vi "复材超声C扫缺陷分析评定软件.vi"() -> ()   [LabVIEW 2018]
doc: "使用该模板构建用户界面事件处理设计模式。将模板应用于对话框及其它用户界面。用户也可创建并执行VI可按照与用户界面事件相同方式处理的用户定义事件。"
uses:
  <vilib>/Utility/NIReport.llb/Report Type.ctl
  <vilib>/addons/_office/_exclsub.llb/font.ctl
  <vilib>/Utility/NIReport.llb/HTML Report Image Alignment.ctl
  <vilib>/Utility/NIReport.llb/Append Report Text (str wrap).vi
  <vilib>/Utility/NIReport.llb/Append Image to Report (path wrap).vi
  <vilib>/addons/_office/word.llb/Word Easy Table (str).vi
  <vilib>/Utility/NIReport.llb/NI_report.lvclass
  <vilib>/vision/NI_Vision_Development_Module.lvlib
  <vilib>/Utility/NIReport.llb/Word/NI_Word.lvclass
  <vilib>/addons/_office/NI_ReportGenerationToolkit.lvlib
  <vilib>/Utility/NIReport.llb/NI_ReportGenerationCore.lvlib
panel:
  in  "删除完成 2":bool caption="定量分析"
  in  "标注完成":bool caption="定量分析"
  in  "删除标注":bool caption="定量分析"
  out "输入的灰度阈值":dbl caption="值"
  out "反射图原始路径":path
  out "穿透图原始路径":path
  out "ROImask":T1(plugin-control)
  in  "Operation 2":enum16{"overlay rectangle"}(ring)
  out "模式选择":u16(ring) items=["只读穿透图", "穿透图和反射图结合"]
  out "添加的路径":path
  out "连接的字符串 2":string
  out "临界面积百分比值":dbl
  out "临界Z值":i32
  out "标注后的图片路径":path
  out "弥散类检测结果合并":string[][](table)
  out "分层类检测结果合并":string[][](table)
  out "弥散类检测结果":string[][](table)
  out "分层类检测结果":string[][](table)
  out "部位信息":string[](array[string])=["", "34.500000", "32.500000", "1121", "34", "54.955926", "分层类", "不合格", ""]
  out "连接的字符串":string
  in  "完成标注":bool caption="定量分析"
  out "框数":dbl
  in  "Operation":enum16{"overlay rectangle"}(ring)
  out "自定义字体":T2={"Desired Font (Application)"=enum."Application Font", "[User-specified Font]"={"Font Name"="", "Size"=12, "Strikeout?"=FALSE, "Italic?"=FALSE, "Underline?"=FALSE, "Outline?"=FALSE, "Shadow?"=FALSE, "Bold?"=FALSE, "Rotation Angle"=0.0}, "Horizontal Alignment"=0, "Vertical Alignment"=0} {"Horizontal Alignment" items=["Left", "Center", "Right"]; "Vertical Alignment" items=["Bottom", "Top", "Baseline"]}
  out "框组":T3(array[cluster])
  out "质量等级":string
  out "灰度阈值":dbl
  in  "stop":bool caption="停止"
  in  "导入图像":bool caption="导入图片"
  in  "图像预处理":bool
  in  "自定义色彩":bool
  in  "开始标注":bool caption="定量分析"
  in  "查看标注":bool caption="辅助定性分析"
  in  "生成评定结果":bool caption="生成原始记录"
  in  "?":enum32{"穿透图", "反射图"}(tab)
  out "穿透图":T1(plugin-control)
  out "反射图":T1(plugin-control)
  out "产品规格":cluster{"产品长度（周长）（mm）":dbl, "产品宽度（母线长）（mm）":dbl}
  out "图像分辨率":T4
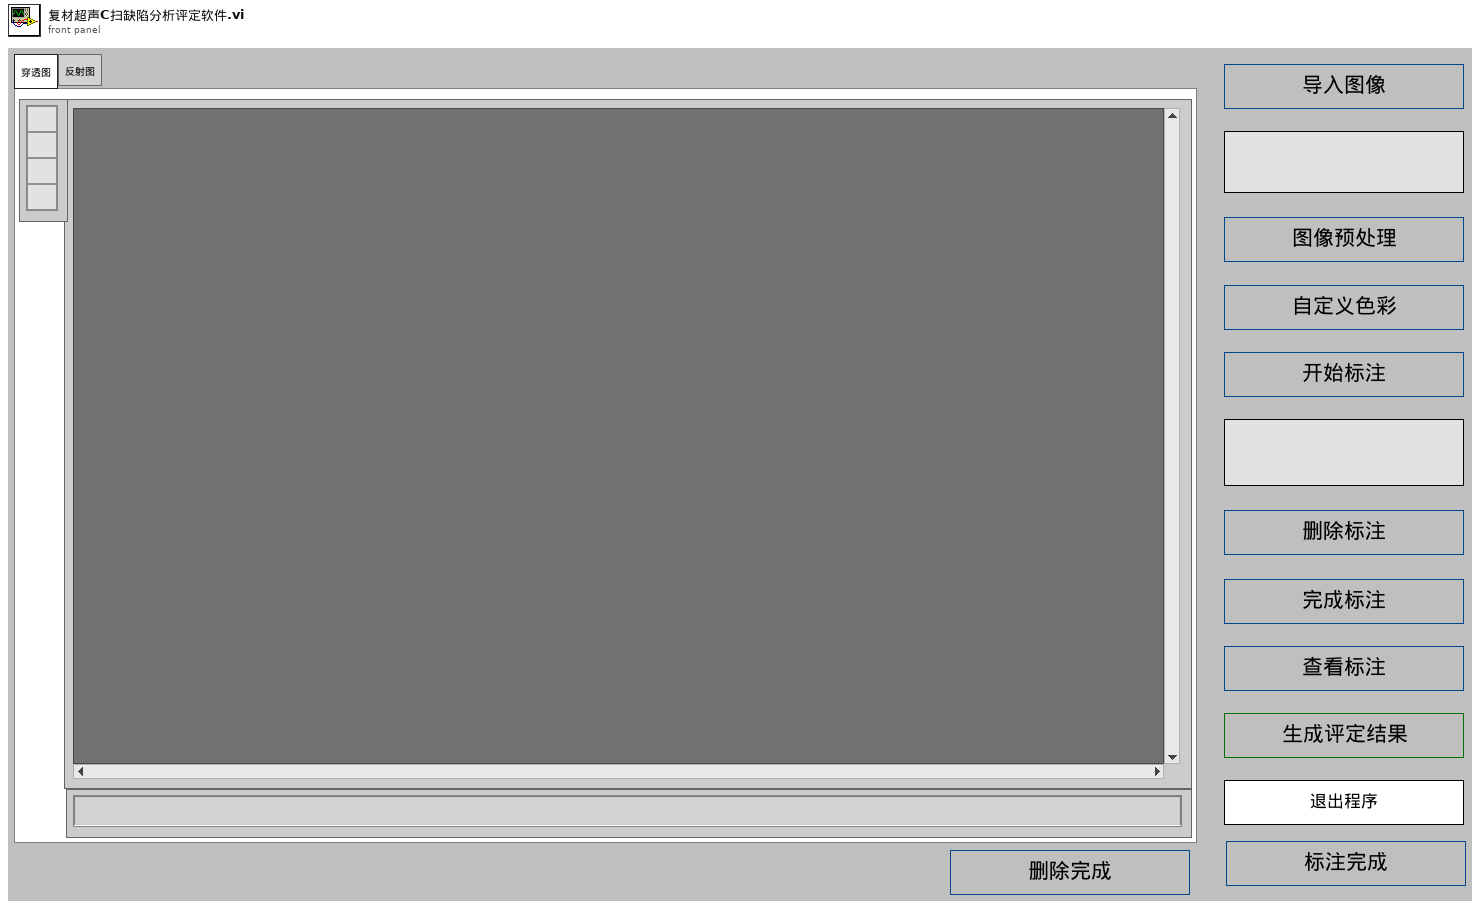
[diagram p1: front panel]
types:
  T1 = typedef "IMAQ Image.ctl" = refnum<image>
  T2 = cluster{"Desired Font (Application)":enum16{"User-specified Font", "Application Font", "System Font", "Dialog Font"}, "[User-specified Font]":cluster{"Font Name":string, "Size":i16, "Strikeout?":bool, "Italic?":bool, "Underline?":bool, "Outline?":bool, "Shadow?":bool, "Bold?":bool, "Rotation Angle":dbl}, "Horizontal Alignment":i16, "Vertical Alignment":i16}
  T3 = cluster{"Global Rectangle":i32[], "Contours":cluster{"Contour Type":u32, "ROI Type":u32, "Points":i32[]}[]}[]
  T4 = cluster{"图像X向分辨率（mm/像素）":dbl, "图像Y向分辨率（mm/像素）":dbl}
  T5 = cluster{"Zoom Tool":bool, "Selection Tool":bool, "Pan Tool":bool, "Point Tool":bool, "Line Tool":bool, "Rectangle Tool":bool, "Rotated Rectangle Tool":bool, "Polyline Tool":bool, "Polygon Tool":bool, "Freehand Tool":bool, "Closed Freehand Tool":bool, "Ellipse Tool":bool, "Annulus Tool":bool}
  T6 = enum32{"Invalid", "Standard", "Closed", "Hidden", "Minimized", "Maximized"}
  T7 = enum32{"Linear", "Log", "Exp", "Square", "Square root", "Power X", "Power 1/X"}
  T8 = enum32{"Gray", "Binary", "Gradient", "Rainbow", "Temperature"}
  T9 = enum16{"initial", "wait", "status1", "status2", "exit"}
  T10 = enum16{"maximized", "minimized", "normal", "no change"}
  T11 = typedef "NI_ReportGenerationCore.lvlib/Report Type.ctl" = enum16{"HTML", "Word", "Excel"}
  T12 = typedef "NI_ReportGenerationCore.lvlib/HTML Report Image Alignment.ctl" = enum16{"(default)", "LEFT", "RIGHT", "TOP", "TEXTTOP", "MIDDLE", "ABSMIDDLE", "BASELINE", "BOTTOM", "ABSBOTTOM"}
  T13 = cluster{"position (Excel)":cluster{"row":i32, "column":i32}, "name (Excel)":string, "bookmark (Word)":string}
  T14 = cluster{"position (excel)":cluster{"row":i32, "column":i32}, "name (excel)":string, "bookmark (word)":string}
  T15 = typedef "NI_ReportGenerationToolkit.lvlib/font.ctl" = cluster{"font name":string, "font size":dbl, "bold":u16, "italic":u16, "underline":u16, "strike through":u16, "font color":u32}
  T16 = typedef "Image Type" = u32
  T17 = cluster{"Red (or Hue) value":u8, "Green (or Sat) value":u8, "Blue (or Light or Val) value":u8}[]
  T18 = cluster{"Global Rectangle":i32[], "Contours":cluster{"Contour Type":u32, "ROI Type":u32, "Points":i32[]}[]}
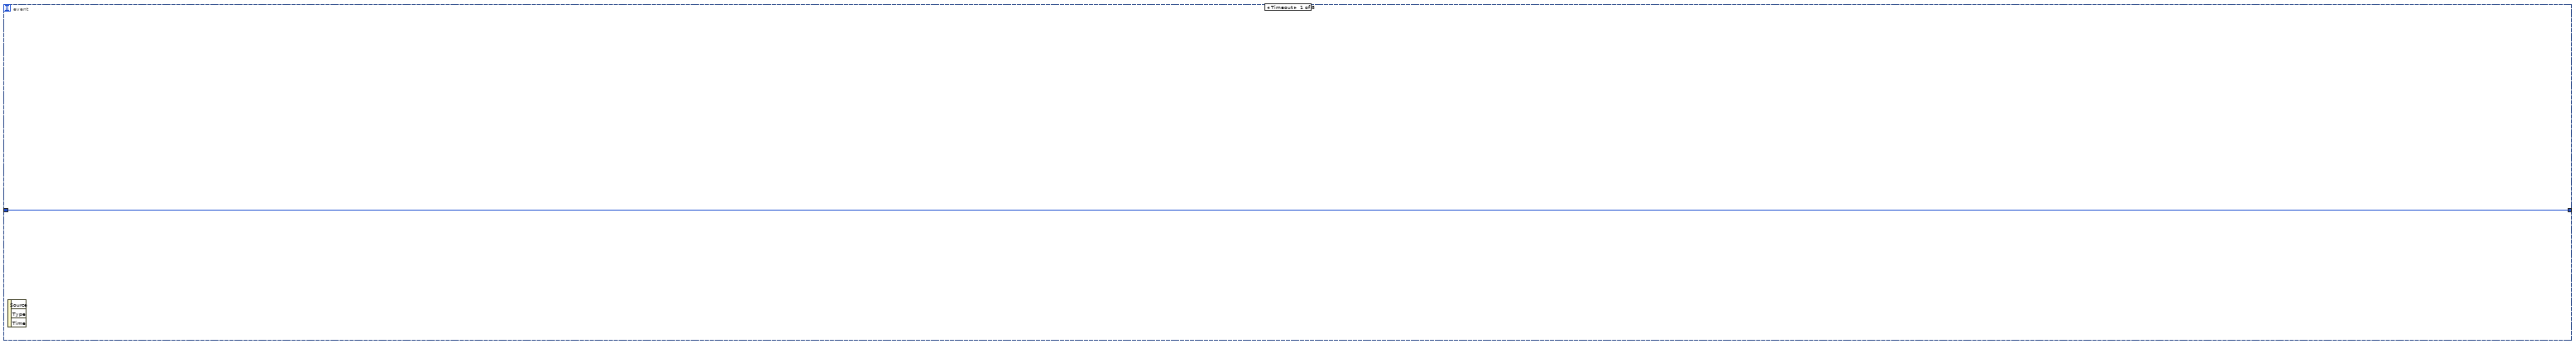
[diagram p3: hidden frame]
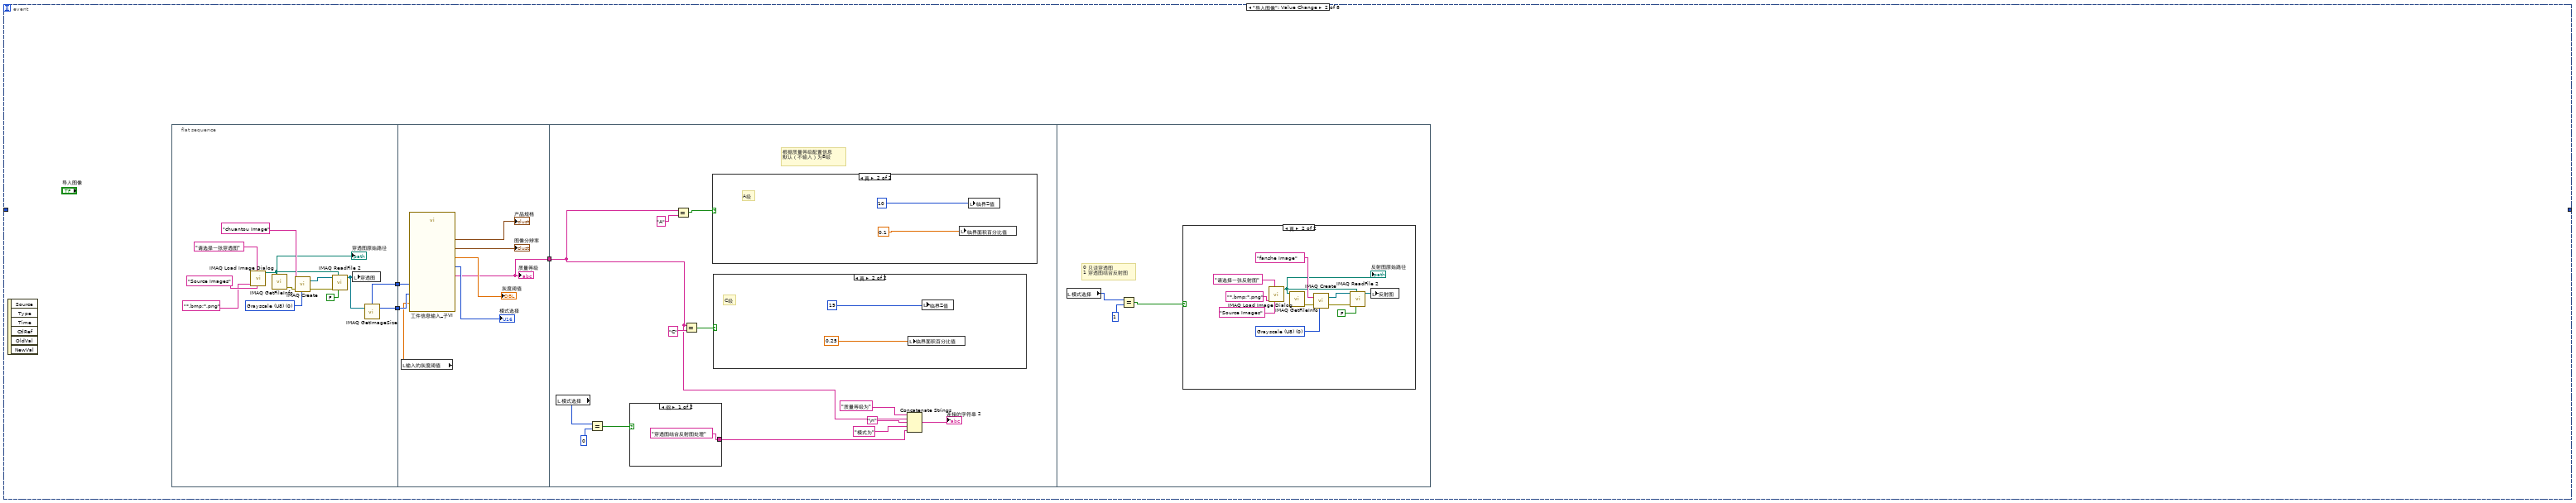
[diagram p4: hidden frame]
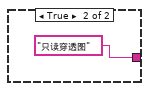
[diagram p5: hidden frame]
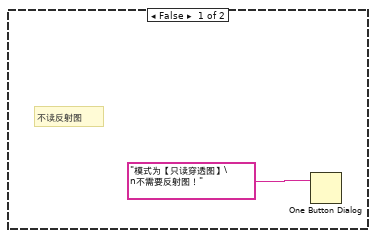
[diagram p8: hidden frame]
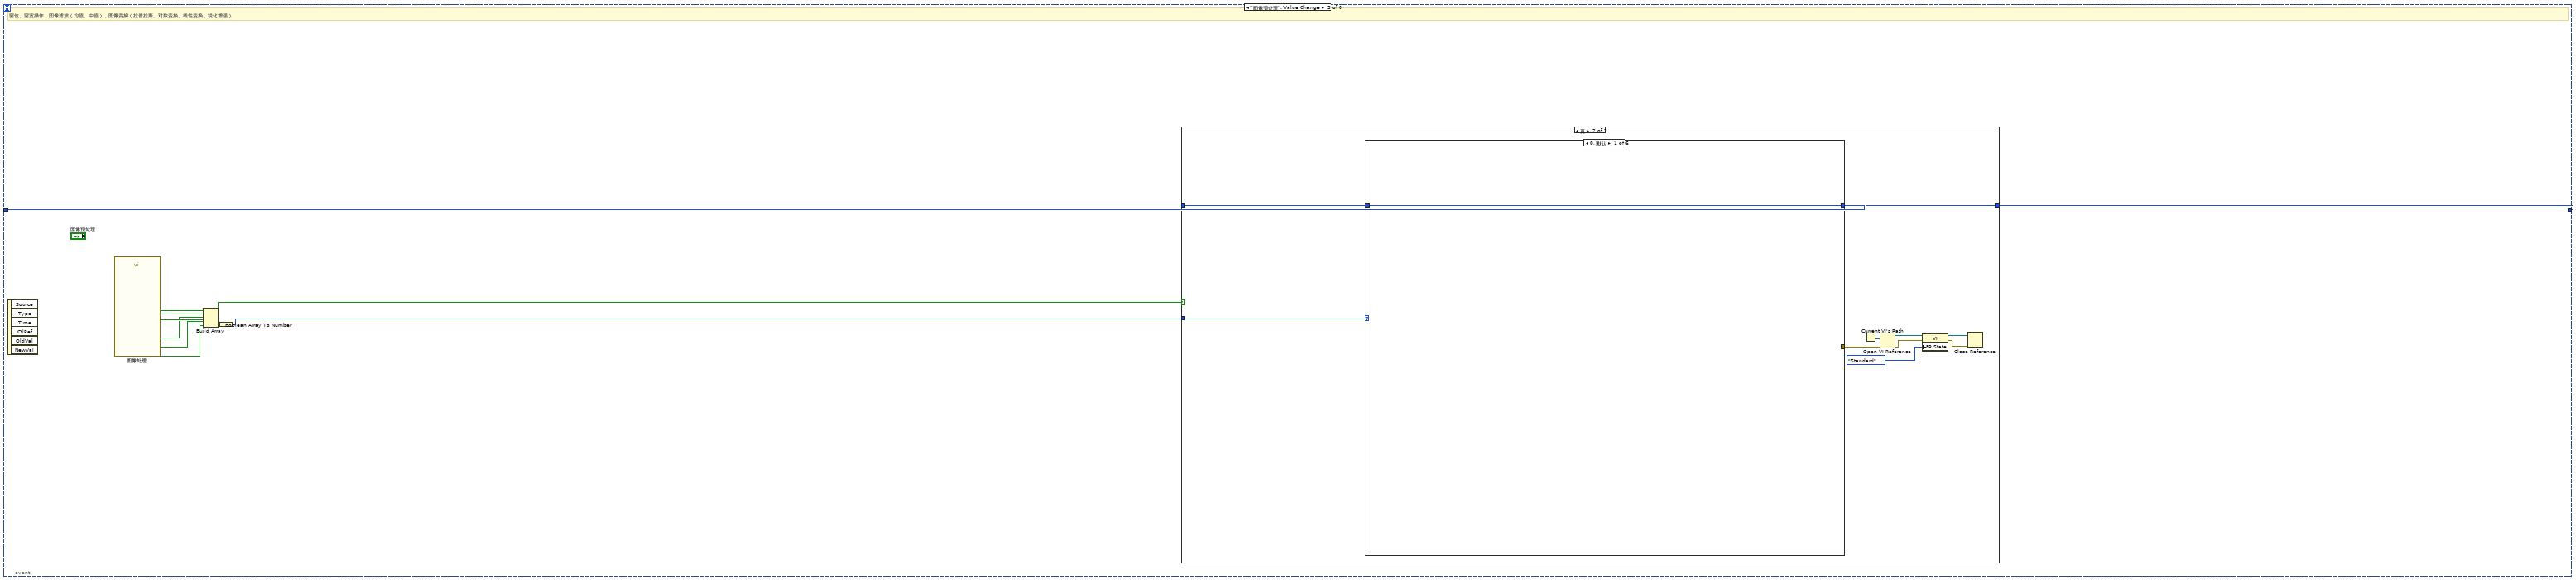
[diagram p9: hidden frame]
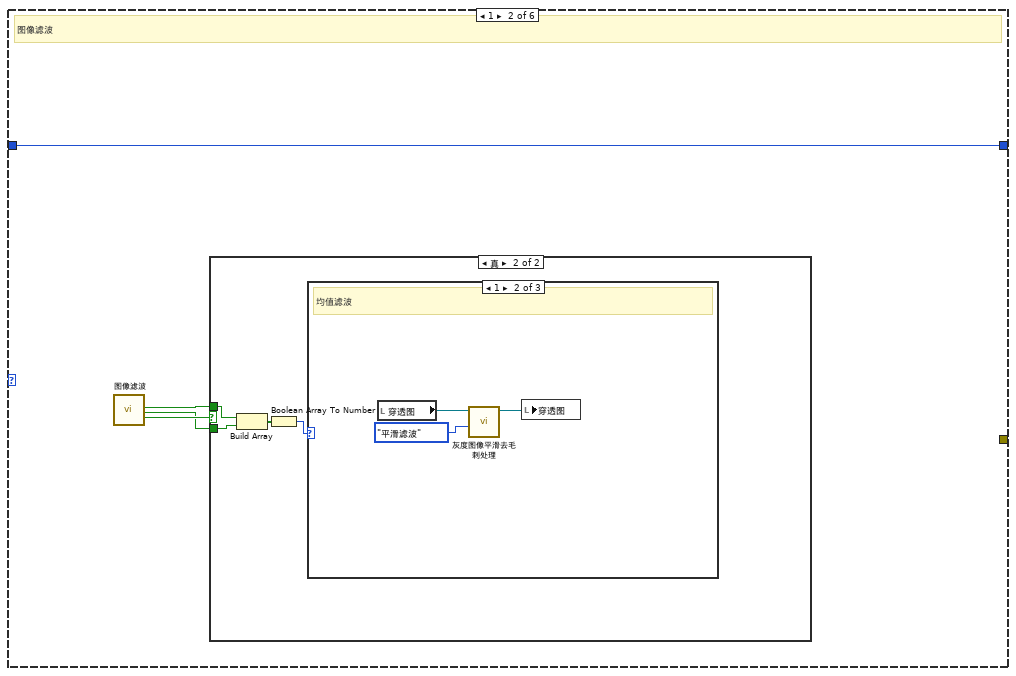
[diagram p11: hidden frame]
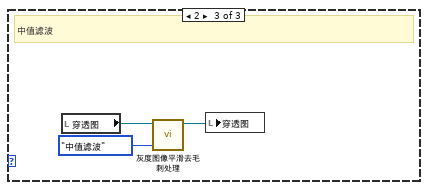
[diagram p14: hidden frame]
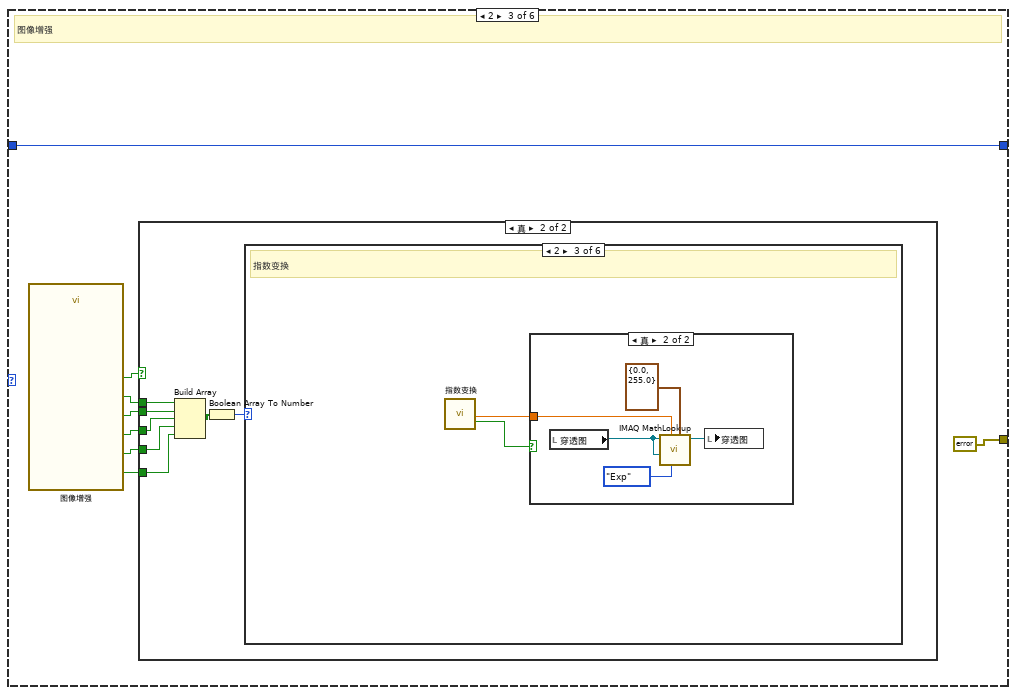
[diagram p15: hidden frame]
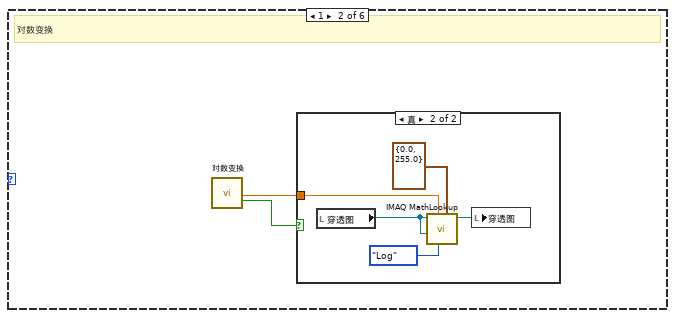
[diagram p18: hidden frame]
diagram:
  w12 = u16 0 items=["只读穿透图", "穿透图和反射图结合"] ("模式选择")
  w1 = FALSE ("查看标注")
  w17 = u32 0 items=["Grayscale", "Binary", "Gradient", "Rainbow", "Temperature", "User Defined", "Binary 16 Bit", "Gradient 16 Bit", "Rainbow 16 Bit", "Temperature 16 Bit", "User Defined 16 Bit"] ("Palette:Palette Type")
  w21 = TRUE ("Zoom to Fit Mode")
  w24 = u32 0 items=["Grayscale", "Binary", "Gradient", "Rainbow", "Temperature", "User Defined", "Binary 16 Bit", "Gradient 16 Bit", "Rainbow 16 Bit", "Temperature 16 Bit", "User Defined 16 Bit"] ("Palette:Palette Type")
  # "默认B级作为评判标准"
  n1 = flat-sequence {
    tunnel: [w28] -> w9
    tunnel: [w27] -> w8
    tunnel: [w26] -> w3
    tunnel: w9 -> [w31]
    tunnel: w8 -> [w32]
    tunnel: [w32] -> w7
    tunnel: [w31] -> w6
    tunnel: [w30] -> w4
    tunnel: w7 -> [w36]
    tunnel: w6 -> [w35]
    tunnel: [w34] -> w5
    frame #0 {
      w27 = "复材分析评定软件" ("section")
      w28 = "判定阈值配置" ("文件名称")
      n2 = call "ini配置文件读取（DBL）.vi"("key"="Z值", "section"=w27, "文件名称"=w28) -> ("value"=w26:dbl)  [unwired: 8 in]
    }
    frame #1 {
      n3 = call "ini配置文件读取（DBL）.vi"("key"="弥散性缺陷阈值", "section"=w32, "文件名称"=w31) -> ("value"=w30:dbl)  [unwired: 8 in]
    }
    frame #2 {
      n4 = call "ini配置文件读取（DBL）.vi"("key"="灰度阈值", "section"=w36, "文件名称"=w35) -> ("value"=w34:dbl)  [unwired: 8 in]
    }
  }
  n5 = To Long Integer(number=w3) -> (32bit integer=→"临界Z值":i32)
  n6 = property on="穿透图" class="ImageControl"("Palette Type"=w24, "ROI Tool Buttons Visible"=T5 {"Zoom Tool"=TRUE, "Selection Tool"=TRUE, "Pan Tool"=TRUE, "Point Tool"=FALSE, "Line Tool"=FALSE, "Rectangle Tool"=TRUE, "Rotated Rectangle Tool"=FALSE, "Polyline Tool"=FALSE, "Polygon Tool"=FALSE, "Freehand Tool"=FALSE, "Closed Freehand Tool"=FALSE, "Ellipse Tool"=FALSE, "Annulus Tool"=FALSE} ("ROI Tool Buttons Visible:All Elements")) -> ()  [unwired: 2 in, 2 out]
  n7 = property on="反射图" class="ImageControl"("Palette Type"=w17, "ROI Tool Buttons Visible"=T5 {"Zoom Tool"=TRUE, "Selection Tool"=TRUE, "Pan Tool"=TRUE, "Point Tool"=FALSE, "Line Tool"=FALSE, "Rectangle Tool"=TRUE, "Rotated Rectangle Tool"=FALSE, "Polyline Tool"=FALSE, "Polygon Tool"=FALSE, "Freehand Tool"=FALSE, "Closed Freehand Tool"=FALSE, "Ellipse Tool"=FALSE, "Annulus Tool"=FALSE} ("ROI Tool Buttons Visible:All Elements")) -> ()  [unwired: 2 in, 2 out]
  n8 = local write "标注后的图片路径"(path "" ("标注后的图片路径")) -> ()
  n9 = local write "连接的字符串 2"("（配置信息）" ("连接的字符串 2")) -> ()
  n10 = local write "连接的字符串"("（标注信息）" ("连接的字符串")) -> ()
  n11 = property on="穿透图" class="ImageControl"("Zoom to Fit Mode"=w21) -> ()  [unwired: 2 in, 2 out]
  n12 = property on="反射图" class="ImageControl"("Zoom to Fit Mode"=w21) -> ()  [unwired: 2 in, 2 out]
  n13 = local write "删除标注"(w1) -> ()
  n14 = local write "查看标注"(w1) -> ()
  n15 = local write "模式选择"(w12) -> ()
  n16 = local write "stop"(w1) -> ()
  n17 = local write "完成标注"(w1) -> ()
  n18 = while {
    shift-right: [w38] -> _
    shift-left: 0 -> [w39]
    stop <- w41 stop-if-true
    n19 = event shown="[4] \"开始标注\": 鼠标按下" {
      selector: _ -> [_ _ _ _ _ _ _ _]
      dyn-events: _ -> [_ _ _ _ _ _ _ _]
      timeout: 100 -> [_ _ _ _ _ _ _ _]
      tunnel: [_ _ _ _ _ _ _ w798] -> w41
      tunnel: w39 -> [w42 _ w102 w240 _ _ w637 _]
      tunnel: [w42 _ w101 w240 _ _ w637 0] -> w38
      event Timeout {
        n20 = event-data() -> ()  [unwired: 1 in, 3 out]
      }
      event "导入图像": Value Change {
        n21 = event-data() -> ()  [unwired: 1 in, 6 out]
        n22 = flat-sequence {
          tunnel: [w47] -> w44
          tunnel: [w46] -> w43
          tunnel: [w62] -> w45
          tunnel: w44 -> [w61]
          tunnel: w43 -> [w60]
          tunnel: w45 -> [w71]
          frame #0 {
            w50 = T16 0 items=["Grayscale (U8)", "Grayscale (I16)", "Grayscale (SGL)", "Complex (CSG)", "RGB (U32)", "HSL (U32)", "RGB (U64)", "Grayscale (U16)"] ("Image Type")
            n23 = call "IMAQ Load Image Dialog"("Pattern Label"="Source Images", "Prompt"="请选择一张穿透图" ("prompt"), "Pattern"="*.bmp;*.png") -> ("Path"=w49:path)  [unwired: 6 in, 2 out]
            "穿透图原始路径" <- w49
            n24 = call "IMAQ GetFileInfo"("File Path"=w49) -> ("error out"=w53:errorcluster)  [unwired: 4 in, 6 out]
            n25 = call "IMAQ Create"("Image Name"="chuantou Image", "Image Type"=w50, "error in (no error)"=w53) -> ("New Image"=w54:T1, "error out"=w55:errorcluster)  [unwired: 2 in]
            n26 = call "IMAQ ReadFile 2"("Use File Path Image Type"=FALSE, "File Path"=w49, "error in (no error)"=w55, "Image"=w54) -> ("Image Out"=w48:T1)  [unwired: 3 in, 4 out]
            n27 = local write "穿透图"(w48) -> ()
            n28 = call "IMAQ GetImageSize"("Image"=w48) -> ("Y Resolution"=w46:i32, "X Resolution"=w47:i32)  [unwired: 3 in, 1 out]
          }
          frame #1 {
            n29 = local read "输入的灰度阈值"() -> (w59:dbl)
            n30 = call "工件信息输入_子VI.vi"("Y Resolution"=w60, "X Resolution"=w61, "输入的灰度阈值"=w59) -> ("质量等级"=w62:string, "模式选择"=→"模式选择":u16, "灰度阈值"=→"灰度阈值":dbl, "产品规格"=→"产品规格":cluster{"产品长度（周长）（mm）":dbl, "产品宽度（母线长）（mm）":dbl}, "图像分辨率"=→"图像分辨率":T4)  [unwired: 3 in]
            "质量等级" <- w62
          }
          frame #2 {
            # "根据质量等级配置信息\n默认（不输入）为B级"
            n31 = local read "模式选择"() -> (w69:u16)
            n32 = Equal?(x=w69, y=u16 0) -> (x = y?=w68:bool)
            n33 = case shown="假" w68 {
              tunnel: ["穿透图结合反射图处理" ("字符串") "只读穿透图" ("字符串")] -> w67
              frame False {
              }
              frame True {
              }
            }
            n34 = Equal?(x=w71, y="A") -> (x = y?=w74:bool)
            n35 = Equal?(x=w71, y="C") -> (x = y?=w75:bool)
            n36 = case shown="真" w74 {
              frame False {
              }
              frame True {
                # "A级"
                n37 = local write "临界面积百分比值"(0.1 ("临界面积百分比值")) -> ()
                n38 = local write "临界Z值"(10 ("临界Z值")) -> ()
              }
            }
            n39 = case shown="真" w75 {
              frame False {
              }
              frame True {
                # "C级"
                n40 = local write "临界面积百分比值"(0.25 ("临界面积百分比值")) -> ()
                n41 = local write "临界Z值"(19 ("临界Z值")) -> ()
              }
            }
            n42 = Concatenate Strings("质量等级为" ("字符串"), w71, "\n", "模式为" ("字符串"), w67) -> (→"连接的字符串 2":string)
          }
          frame #3 {
            # "0 只读穿透图\n1 穿透图结合反射图"
            n43 = local read "模式选择"() -> (w87:u16)
            n44 = Equal?(x=w87, y=u16 1) -> (x = y?=w86:bool)
            n45 = case shown="真" w86 {
              frame False {
                # "不读反射图"
                n46 = One Button Dialog(message="模式为【只读穿透图】\n不需要反射图！" ("消息")) -> ()  [unwired: 1 in, 1 out]
              }
              frame True {
                w92 = T16 0 items=["Grayscale (U8)", "Grayscale (I16)", "Grayscale (SGL)", "Complex (CSG)", "RGB (U32)", "HSL (U32)", "RGB (U64)", "Grayscale (U16)"] ("Image Type")
                n47 = call "IMAQ Load Image Dialog"("Pattern Label"="Source Images", "Prompt"="请选择一张反射图" ("prompt"), "Pattern"="*.bmp;*.png") -> ("Path"=w91:path)  [unwired: 6 in, 2 out]
                "反射图原始路径" <- w91
                n48 = call "IMAQ GetFileInfo"("File Path"=w91) -> ("error out"=w95:errorcluster)  [unwired: 4 in, 6 out]
                n49 = call "IMAQ Create"("Image Name"="fanshe Image", "Image Type"=w92, "error in (no error)"=w95) -> ("New Image"=w96:T1, "error out"=w97:errorcluster)  [unwired: 2 in]
                n50 = call "IMAQ ReadFile 2"("Use File Path Image Type"=FALSE, "File Path"=w91, "error in (no error)"=w97, "Image"=w96) -> ("Image Out"=w90:T1)  [unwired: 3 in, 4 out]
                n51 = local write "反射图"(w90) -> ()
              }
            }
          }
        }
      }
      event "图像预处理": Value Change {
        # "窗位、窗宽操作，图像滤波（均值、中值），图像变换（拉普拉斯、对数变换、线性变换、锐化增强）"
        n52 = event-data() -> ()  [unwired: 1 in, 6 out]
        n53 = call "图像处理"() -> ("撤销图像处理"=w103:bool, "线性灰度值测量"=w104:bool, "窗位窗宽"=w109:bool, "图像增强"=w105:bool, "图像滤波"=w110:bool, "确定"=w106:bool)  [unwired: 13 in, 1 out]
        n54 = Build Array(w110, w105, w109, w104, w103) -> (w108:bool[])
        n55 = Boolean Array To Number(Boolean array=w108) -> (number=w107:u32)
        n56 = case shown="真" w106 {
          tunnel: w107 -> [_ w121]
          tunnel: w102 -> [w111 w113]
          tunnel: [w111 w112] -> w101
          frame False {
          }
          frame True {
            n57 = case shown="0, 默认" w121 {
              tunnel: [_ _ errorcluster {"status"=FALSE, "code"=0, "source"=""} ("错误输入（无错误）") _ _ _] -> w114
              tunnel: w113 -> [w122 w123 w137 w186 w209 w231]
              tunnel: [w122 w123 w137 w186 w209 w231] -> w112
              frame 0, Default {
              }
              frame 1 {
                # "图像滤波"
                n58 = call "图像滤波"() -> ("均值滤波"=w125:bool, "中值滤波"=w124:bool, "确定"=w126:bool)  [unwired: 16 in, 1 out]
                n59 = case shown="真" w126 {
                  tunnel: w125 -> [_ w129]
                  tunnel: w124 -> [_ w128]
                  frame False {
                  }
                  frame True {
                    n60 = Build Array(w129, w128) -> (w130:bool[])
                    n61 = Boolean Array To Number(Boolean array=w130) -> (number=w127:u32)
                    n62 = case shown="1" w127 {
                      frame 0, Default {
                      }
                      frame 1 {
                        # "均值滤波"
                        n63 = local read "穿透图"() -> (w133:T1)
                        n64 = call "灰度图像平滑去毛刺处理.vi"("滤波方法选择"=enum16{"中值滤波", "平滑滤波"}."平滑滤波", "Image"=w133) -> ("Image Out"=w132:T1)  [unwired: 9 in]
                        n65 = local write "穿透图"(w132) -> ()
                      }
                      frame 2 {
                        # "中值滤波"
                        n66 = local read "穿透图"() -> (w136:T1)
                        n67 = call "灰度图像平滑去毛刺处理.vi"("滤波方法选择"=enum16{"中值滤波", "平滑滤波"}."中值滤波", "Image"=w136) -> ("Image Out"=w135:T1)  [unwired: 9 in]
                        n68 = local write "穿透图"(w135) -> ()
                      }
                    }
                  }
                }
              }
              frame 2 {
                # "图像增强"
                n69 = call "图像增强"() -> ("幂变换"=w139:bool, "阈值变换"=w140:bool, "高斯变换"=w141:bool, "指数变换"=w142:bool, "对数变换"=w143:bool, "确定"=w144:bool)  [unwired: 13 in, 1 out]
                n70 = case shown="真" w144 {
                  tunnel: w143 -> [_ w149]
                  tunnel: w142 -> [_ w148]
                  tunnel: w141 -> [_ w147]
                  tunnel: w140 -> [_ w146]
                  tunnel: w139 -> [_ w145]
                  frame False {
                  }
                  frame True {
                    n71 = Build Array(w149, w148, w147, w146, w145) -> (w151:bool[])
                    n72 = Boolean Array To Number(Boolean array=w151) -> (number=w150:u32)
                    n73 = case shown="2" w150 {
                      frame 0, Default {
                      }
                      frame 1 {
                        # "对数变换"
                        n74 = call "对数变换"() -> ("变换系数K"=w152:dbl, "确定"=w153:bool)  [unwired: 17 in, 1 out]
                        n75 = case shown="真" w153 {
                          tunnel: w152 -> [_ w154]
                          frame False {
                          }
                          frame True {
                            n76 = local read "穿透图"() -> (w158:T1)
                            n77 = call "IMAQ MathLookup"("Range"=cluster{"Minimum":sgl, "Maximum":sgl} {"Minimum"=0.0, "Maximum"=255.0}, "Operator"=T7."Log", "X Value"=w154, "Image Dst"=w158, "Image Src"=w158) -> ("Image Dst Out"=w156:T1)  [unwired: 5 in, 1 out]
                            n78 = local write "穿透图"(w156) -> ()
                          }
                        }
                      }
                      frame 2 {
                        # "指数变换"
                        n79 = call "指数变换"() -> ("变换系数K"=w159:dbl, "确定"=w160:bool)  [unwired: 17 in, 1 out]
                        n80 = case shown="真" w160 {
                          tunnel: w159 -> [_ w161]
                          frame False {
                          }
                          frame True {
                            n81 = local read "穿透图"() -> (w165:T1)
                            n82 = call "IMAQ MathLookup"("Range"=cluster{"Minimum":sgl, "Maximum":sgl} {"Minimum"=0.0, "Maximum"=255.0}, "Operator"=T7."Exp", "X Value"=w161, "Image Dst"=w165, "Image Src"=w165) -> ("Image Dst Out"=w163:T1)  [unwired: 5 in, 1 out]
                            n83 = local write "穿透图"(w163) -> ()
                          }
                        }
                      }
                      frame 4 {
                        w171 = u16 4 items=["Gradient"=1, "Laplacian"=2, "Smoothing"=3, "Gaussian"=4] ("Kernel Family")
                        # "高斯斯变换"
                        n84 = local read "穿透图"() -> (w168:T1)
                        n85 = call "IMAQ GetKernel"("Kernel Family"=w171, "Kernel Size (3,5,...)"=3) -> ("Kernel"=w169:sgl[][], "Divider"=w166:sgl)  [unwired: 6 in, 2 out]
                        n86 = call "IMAQ Convolute"("Kernel"=w169, "Divider (kernel sum)"=w166, "Image Dst"=w168, "Image Src"=w168) -> ("Image Dst Out"=w167:T1)  [unwired: 6 in, 1 out]
                        n87 = local write "穿透图"(w167) -> ()
                      }
                      frame 8 {
                        # "阈值变换"
                        n88 = call "阈值范围选择子VI.vi"() -> ("阈值范围"=w172:cluster{"Lower value":sgl, "Upper value":sgl}, "确定执行"=w173:bool)  [unwired: 10 in]
                        n89 = case shown="真" w173 {
                          tunnel: w172 -> [_ w175]
                          frame False {
                          }
                          frame True {
                            n90 = local read "穿透图"() -> (w178:T1)
                            n91 = call "IMAQ Threshold"("Replace Value"=sgl 255.0, "Keep/Replace Value (Replace)"=TRUE, "Range"=w175, "Image Dst"=w178, "Image Src"=w178) -> ("Image Dst Out"=w177:T1)  [unwired: 5 in, 1 out]
                            n92 = local write "穿透图"(w177) -> ()
                          }
                        }
                      }
                      frame 16 {
                        # "幂变换"
                        n93 = call "幂变换"() -> ("变换系数K"=w179:dbl, "确定"=w180:bool)  [unwired: 17 in, 1 out]
                        n94 = case shown="真" w180 {
                          tunnel: w179 -> [_ w181]
                          frame False {
                          }
                          frame True {
                            n95 = local read "穿透图"() -> (w185:T1)
                            n96 = call "IMAQ MathLookup"("Range"=cluster{"Minimum":sgl, "Maximum":sgl} {"Minimum"=0.0, "Maximum"=255.0}, "Operator"=T7."Power 1/X", "X Value"=w181, "Image Dst"=w185, "Image Src"=w185) -> ("Image Dst Out"=w183:T1)  [unwired: 5 in, 1 out]
                            n97 = local write "穿透图"(w183) -> ()
                          }
                        }
                      }
                    }
                  }
                }
              }
              frame 4 {
                # "窗位窗宽"
                n98 = Two Button Dialog(message="确定进行窗位窗宽操作？" ("消息")) -> (T button?=w188:bool)  [unwired: 2 in]
                n99 = case shown="真" w188 {
                  frame False {
                  }
                  frame True {
                    n100 = property on="穿透图" class="ImageControl"() -> (error out=w190:errorcluster, "Palette Type"=w197:u32)  [unwired: 2 in, 1 out]
                    n101 = Current VI's Path() -> (path=w192:path)
                    n102 = Open VI Reference(vi path=w192, error in (no error)=w190) -> (vi reference=w193:refnum<vi>, error out=w195:errorcluster)  [unwired: 4 in]
                    n103 = case shown="4" w197 {
                      tunnel: [w200 w202 w204 w206 w208] -> w198
                      frame 0, Default {
                        # "灰度"
                        n104 = call "IMAQ GetPalette"("Palette Number (gray)"=T8."Gray") -> ("Color Palette"=w200:cluster{"Red":u8, "Green":u8, "Blue":u8}[])  [unwired: 4 in, 1 out]
                      }
                      frame 2 {
                        # "梯度"
                        n105 = call "IMAQ GetPalette"("Palette Number (gray)"=T8."Gradient") -> ("Color Palette"=w202:cluster{"Red":u8, "Green":u8, "Blue":u8}[])  [unwired: 4 in, 1 out]
                      }
                      frame 3 {
                        # "彩虹"
                        n106 = call "IMAQ GetPalette"("Palette Number (gray)"=T8."Rainbow") -> ("Color Palette"=w204:cluster{"Red":u8, "Green":u8, "Blue":u8}[])  [unwired: 4 in, 1 out]
                      }
                      frame 4 {
                        # "温度"
                        n107 = call "IMAQ GetPalette"("Palette Number (gray)"=T8."Temperature") -> ("Color Palette"=w206:cluster{"Red":u8, "Green":u8, "Blue":u8}[])  [unwired: 4 in, 1 out]
                      }
                      frame 5 {
                        # "自定义"
                        n108 = property on="穿透图" class="ImageControl"() -> ("User Palette"=w208:cluster{"Red":u8, "Green":u8, "Blue":u8}[])  [unwired: 2 in, 2 out]
                      }
                    }
                    n109 = property class="VI"(reference=w193, error in=w195, "FP.State"=T6."Hidden" ("前面板窗口:状态")) -> (reference out=w194:refnum<vi>, error out=w196:errorcluster)
                    n110 = Close Reference(reference=w194, error in (no error)=w196) -> ()  [unwired: 1 out]
                    n111 = local read "穿透图"() -> (w189:T1)
                    n112 = call "窗位窗宽调整子VI.vi"("Image in"=w189, "Palette:User Palette"=w198, "Palette:Palette Type"=w197) -> ("Image out"=w199:T1)  [unwired: 8 in]
                    n113 = local write "穿透图"(w199) -> ()
                  }
                }
              }
              frame 8 {
                # "查看线灰度值曲线，用于精确测量"
                n114 = Current VI's Path() -> (path=w216:path)
                n115 = Open VI Reference(vi path=w216) -> (vi reference=w215:refnum<vi>, error out=w213:errorcluster)  [unwired: 5 in]
                n116 = property class="VI"(reference=w215, error in=w213, "FP.State"=T6."Hidden" ("前面板窗口:状态")) -> (reference out=w214:refnum<vi>, error out=w212:errorcluster)
                n117 = Close Reference(reference=w214, error in (no error)=w212) -> (error out=w210:errorcluster)
                n118 = case shown="无错误" w210 {
                  frame No Error {
                    n119 = property on="穿透图" class="ImageControl"() -> ("Palette Type"=w218:u32)  [unwired: 2 in, 2 out]
                    n120 = case shown="2" w218 {
                      tunnel: [w221 w223 w225 w227 w229] -> w217
                      frame 0, Default {
                        # "灰度"
                        n121 = call "IMAQ GetPalette"("Palette Number (gray)"=T8."Gray") -> ("Color Palette"=w221:cluster{"Red":u8, "Green":u8, "Blue":u8}[])  [unwired: 4 in, 1 out]
                      }
                      frame 2 {
                        # "梯度"
                        n122 = call "IMAQ GetPalette"("Palette Number (gray)"=T8."Gradient") -> ("Color Palette"=w223:cluster{"Red":u8, "Green":u8, "Blue":u8}[])  [unwired: 4 in, 1 out]
                      }
                      frame 3 {
                        # "彩虹"
                        n123 = call "IMAQ GetPalette"("Palette Number (gray)"=T8."Rainbow") -> ("Color Palette"=w225:cluster{"Red":u8, "Green":u8, "Blue":u8}[])  [unwired: 4 in, 1 out]
                      }
                      frame 4 {
                        # "温度"
                        n124 = call "IMAQ GetPalette"("Palette Number (gray)"=T8."Temperature") -> ("Color Palette"=w227:cluster{"Red":u8, "Green":u8, "Blue":u8}[])  [unwired: 4 in, 1 out]
                      }
                      frame 5 {
                        # "自定义"
                        n125 = property on="穿透图" class="ImageControl"() -> ("User Palette"=w229:cluster{"Red":u8, "Green":u8, "Blue":u8}[])  [unwired: 2 in, 2 out]
                      }
                    }
                    n126 = local read "穿透图"() -> (w220:T1)
                    n127 = local read "图像分辨率"() -> (w219:T4)
                    n128 = call "线性灰度值曲线查看子VI.vi"("Palette:User Palette"=w217, "图像分辨率"=w219, "Image"=w220) -> ()  [unwired: 9 in]
                  }
                  frame Error {
                  }
                }
              }
              frame 16 {
                # "撤销图像处理，恢复原图"
                n129 = call "IMAQ Create"("Image Name"="P1") -> ("New Image"=w230:T1)  [unwired: 4 in, 1 out]
                n130 = local write "穿透图"(w230) -> ()
              }
            }
            n131 = Current VI's Path() -> (path=w120:path)
            n132 = Open VI Reference(vi path=w120, error in (no error)=w114) -> (vi reference=w119:refnum<vi>, error out=w116:errorcluster)  [unwired: 4 in]
            n133 = property class="VI"(reference=w119, error in=w116, "FP.State"=T6."Standard" ("前面板窗口:状态")) -> (reference out=w117:refnum<vi>, error out=w115:errorcluster)
            n134 = Close Reference(reference=w117, error in (no error)=w115) -> ()  [unwired: 1 out]
          }
        }
      }
      event "自定义色彩": Value Change {
        # "色彩、色阶自定义"
        n135 = event-data() -> ()  [unwired: 1 in, 6 out]
        n136 = call "调色板"() -> ("自定义显示"=w234:bool, "温度显示"=w235:bool, "彩虹显示"=w236:bool, "梯度显示"=w237:bool, "灰度显示"=w238:bool, "确定"=w239:bool)  [unwired: 13 in, 1 out]
        n137 = Build Array(w238, w237, w236, w235, w234) -> (w233:bool[])
        n138 = case shown="真" w239 {
          tunnel: w233 -> [_ w243]
          frame False {
          }
          frame True {
            n139 = Boolean Array To Number(Boolean array=w243) -> (number=w242:u32)
            n140 = case shown="0, 默认" w242 {
              tunnel: [w244 w245 w246 w247 w248 w250] -> w241
              frame 0, Default {
                w244 = u32 0 items=["Grayscale", "Binary", "Gradient", "Rainbow", "Temperature", "User Defined", "Binary 16 Bit", "Gradient 16 Bit", "Rainbow 16 Bit", "Temperature 16 Bit", "User Defined 16 Bit"] ("Palette:Palette Type")
              }
              frame 1 {
                w245 = u32 0 items=["Grayscale", "Binary", "Gradient", "Rainbow", "Temperature", "User Defined", "Binary 16 Bit", "Gradient 16 Bit", "Rainbow 16 Bit", "Temperature 16 Bit", "User Defined 16 Bit"] ("Palette:Palette Type")
                # "灰度"
              }
              frame 2 {
                w246 = u32 2 items=["Grayscale", "Binary", "Gradient", "Rainbow", "Temperature", "User Defined", "Binary 16 Bit", "Gradient 16 Bit", "Rainbow 16 Bit", "Temperature 16 Bit", "User Defined 16 Bit"] ("Palette:Palette Type")
                # "梯度"
              }
              frame 4 {
                w247 = u32 3 items=["Grayscale", "Binary", "Gradient", "Rainbow", "Temperature", "User Defined", "Binary 16 Bit", "Gradient 16 Bit", "Rainbow 16 Bit", "Temperature 16 Bit", "User Defined 16 Bit"] ("Palette:Palette Type")
                # "彩虹"
              }
              frame 8 {
                w248 = u32 4 items=["Grayscale", "Binary", "Gradient", "Rainbow", "Temperature", "User Defined", "Binary 16 Bit", "Gradient 16 Bit", "Rainbow 16 Bit", "Temperature 16 Bit", "User Defined 16 Bit"] ("Palette:Palette Type")
                # "温度"
              }
              frame 16 {
                w250 = u32 5 items=["Grayscale", "Binary", "Gradient", "Rainbow", "Temperature", "User Defined", "Binary 16 Bit", "Gradient 16 Bit", "Rainbow 16 Bit", "Temperature 16 Bit", "User Defined 16 Bit"] ("Palette:Palette Type")
                # "自定义"
                n141 = call "自定义成像色谱20200214.vi"() -> ("Color palette"=w249:T17)  [unwired: 8 in, 1 out]
                n142 = property on="穿透图" class="ImageControl"("User Palette"=w249) -> ()  [unwired: 2 in, 2 out]
              }
            }
            n143 = property on="穿透图" class="ImageControl"("Palette Type"=w241) -> ()  [unwired: 2 in, 2 out]
          }
        }
      }
      event "开始标注": Mouse Down {
        w251 = FALSE ("完成标注")
        # "0 只读穿透图\n1 穿透图和反射图结合"
        # "手动画框ROI，提取框组（坐标）、框数等信息"
        n144 = event-data() -> ()  [unwired: 1 in, 6 out]
        n145 = local read "模式选择"() -> (w252:u16)
        n146 = One Button Dialog(message="开始标注！\n全部标注完成后，\n请点击“完成标注”按钮" ("消息")) -> ()  [unwired: 1 in, 1 out]
        n147 = local write "删除标注"(w251) -> ()
        n148 = local write "完成标注"(w251) -> ()
        n149 = local write "查看标注"(w251) -> ()
        n150 = case shown="0, 默认" w252 {
          tunnel: w251 -> [_ _]
          frame 0, Default {
            # "只对穿透图时画框的分支"
            n151 = while {
              shift-right: [w265] -> _
              shift-left: _ -> [w264]
              tunnel: [w262] -> _
              shift-right: [w256] -> _
              shift-left: T9."initial" -> [w257]
              stop <- w258 stop-if-true
              (unwired) "_" ("名称或相对路径")
              (unwired) ".docx" ("名称或相对路径")
              n152 = local read "穿透图"() -> (w263:T1)
              n153 = property on="穿透图" class="ImageControl"() -> ("ROI"=w259:T18)  [unwired: 2 in, 2 out]
              n154 = case shown="\"status1\"" w257 {
                tunnel: w263 -> [w267 w270 w288 w365 w409]
                tunnel: [w267 w270 w287 w365 w409] -> w262
                tunnel: "Operation 2" -> [_ _ w286 _ _]
                tunnel: [w269 w274 w284 w363 w413] -> w265
                tunnel: w264 -> [w269 w274 w285 w363 w413]
                tunnel: w259 -> [_ _ w283 _ _]
                tunnel: [T9."wait" w271 w282 w361 T9."exit"] -> w256
                tunnel: [FALSE FALSE FALSE ("T button?") FALSE w411] -> w255
                frame "initial", Default {
                }
                frame "wait" {
                  n155 = disable-structure shown="禁用" {
                    frame Disabled {
                      w275 = i32[] [2] items=["No Event"=0, "Click Event"=1, "Draw Event"=2, "Size Event"=4, "Scroll Event"=5, "Double Click Event"=8] ("Which Events")
                      # "循环的方式给输入图像手动画框"
                      n156 = invoke on="穿透图" class="ImageControl" method="Get Last Event"("Which Events"=w275) -> ("Type"=w276:i32)  [unwired: 7 in, 7 out]
                      n157 = Not Equal To 0?(x=w276) -> ()  [unwired: 1 out]
                    }
                    frame Enabled {
                    }
                  }
                  n158 = event shown="[2] \"开始标注\": 鼠标按下" {
                    selector: _ -> [_ _ _ _]
                    dyn-events: _ -> [_ _ _ _]
                    timeout: 50 -> [_ _ _ _]
                    tunnel: [T9."wait" T9."exit" T9."status1" T9."status2"] -> w271
                    event Timeout {
                      n159 = event-data() -> ()  [unwired: 1 in, 3 out]
                    }
                    event "完成标注": Mouse Down {
                      n160 = event-data() -> ()  [unwired: 1 in, 7 out]
                    }
                    event "开始标注": Mouse Down {
                      n161 = event-data() -> ()  [unwired: 1 in, 7 out]
                    }
                    event "删除标注": Mouse Down {
                      n162 = event-data() -> ()  [unwired: 1 in, 7 out]
                    }
                  }
                }
                frame "status1" {
                  n163 = while {
                    tunnel: w286 -> [w297]
                    tunnel: w285 -> [w296]
                    tunnel: [w295] -> w284
                    tunnel: w283 -> [w294]
                    shift-right: [w298] -> w287
                    shift-left: w288 -> [w299]
                    tunnel: [T9."wait"] -> w282
                    stop <- "标注完成" stop-if-true
                    w290 = i32[] [2] items=["No Event"=0, "Click Event"=1, "Draw Event"=2, "Size Event"=4, "Scroll Event"=5, "Double Click Event"=8] ("Which Events")
                    # "循环的方式给输入图像手动画框"
                    n164 = invoke on="穿透图" class="ImageControl" method="Get Last Event"("Which Events"=w290) -> ("Type"=w291:i32)  [unwired: 7 in, 7 out]
                    n165 = Not Equal To 0?(x=w291) -> (x != 0?=w289:bool)
                    n166 = case shown="真" w289 {
                      tunnel: w299 -> [w300 w308]
                      tunnel: [w300 w307] -> w298
                      tunnel: w297 -> [_ w306]
                      tunnel: w296 -> [w301 w305]
                      tunnel: [w301 w304] -> w295
                      tunnel: w294 -> [_ w303]
                      frame False {
                        n167 = Wait (ms)(milliseconds to wait=u32 100 ("等待时间（毫秒）")) -> ()  [unwired: 1 out]
                      }
                      frame True {
                        n168 = case shown="\"overlay rectangle\"" w306 {
                          tunnel: w308 -> [w320]
                          tunnel: [w319] -> w307
                          tunnel: w305 -> [w318]
                          tunnel: [w317] -> w304
                          tunnel: w303 -> [w309]
                          frame "overlay rectangle" {
                            n169 = flat-sequence {
                              tunnel: w320 -> [w321]
                              tunnel: [w321] -> w316
                              tunnel: w309 -> [w324]
                              tunnel: [w324] -> w315
                              tunnel: w318 -> [w323]
                              tunnel: [w322] -> w314
                              tunnel: w316 -> [w333]
                              tunnel: w315 -> [w332]
                              tunnel: w314 -> [w331]
                              tunnel: [w335] -> w313
                              tunnel: [w331] -> w312
                              tunnel: [w328] -> w311
                              tunnel: [w326] -> w310
                              tunnel: w313 -> [w358]
                              tunnel: w312 -> [w357]
                              tunnel: w311 -> [w349]
                              tunnel: w310 -> [w346]
                              tunnel: [w358] -> w319
                              tunnel: [w357] -> w317
                              frame #0 {
                                # "将当前ROI数据存入框组内"
                                n170 = Build Array (concatenate)(w323, w324) -> (w322:T3)
                                n171 = local write "框组"(w322) -> ()
                              }
                              frame #1 {
                                # "在穿透图上画框"
                                # "图层名Group与“框&图层计数”变量同名，\neg：1号框对应group1"
                                # "overlay text在ROI的左上角添加计数显示"
                                # "overlay ROI代表用户手画绿色框的图层添加"
                                n172 = local read "框组"() -> (w338:T3)
                                n173 = Unbundle(w332) -> ("Global Rectangle"=w341:i32[])  [unwired: 1 out]
                                n174 = Array Size(array=w338) -> (size(s)=w326:i32)
                                n175 = Number To Decimal String(number=w326) -> (decimal integer string=w327:string)  [unwired: 1 in]
                                n176 = local write "框数"(w326) -> ()
                                n177 = Index Array(array=w341, index=1 ("索引")) -> (element=w339:i32)
                                n178 = Index Array(array=w341, index=0 ("索引")) -> (element=w340:i32)
                                n179 = Concatenate Strings(w327, "#" ("字符串")) -> (w328:string)
                                n180 = call "IMAQ Overlay ROI"("Group"=w328, "ROI Descriptor"=w332, "Image"=w333) -> ("Image Out"=w342:T1)  [unwired: 7 in, 1 out]
                                n181 = Bundle(w340, w339) -> (w334:cluster{i32, i32})  [unwired: 1 in]
                                n182 = local read "自定义字体"() -> (w330:T2)
                                n183 = call "IMAQ Overlay Text"("Group"=w328, "Text Color (black)"=u32 16711680, "Font, Size & Style"=w330, "String"=w328, "Origin"=w334, "Image"=w342) -> ("Image Out"=w335:T1)  [unwired: 4 in, 1 out]
                              }
                              frame #2 {
                                # "存放部位信息的1D数组，后续生成报告使用"
                                # "0：位于蒙皮部位\n1：位于筋条部位"
                                n184 = call "缺陷部位标注2"() -> ("位于筋条处"=w354:bool, "位于蒙皮处"=w353:bool)  [unwired: 16 in, 2 out]
                                n185 = Build Array(w353, w354) -> (w355:bool[])
                                n186 = Boolean Array To Number(Boolean array=w355) -> (number=w356:u32)
                                n187 = case shown="1, 默认" w356 {
                                tunnel: ["蒙皮处" ("t") "筋条处" ("t")] -> w344
                                frame 1, Default {
                                }
                                frame 2 {
                                }
                                }
                                n188 = local read "部位信息"() -> (w348:string[])
                                n189 = Decrement(x=w346) -> (x-1=w345:i32)
                                n190 = Insert Into Array(array=w348, index=w345, new element=w344) -> (w347:string[])
                                n191 = Concatenate Strings("框号为" ("字符串"), w349, "\n", "类别为" ("字符串"), w344) -> (w343:string)
                                n192 = local write "连接的字符串"(w343) -> ()
                                n193 = local write "部位信息"(w347) -> ()
                              }
                            }
                          }
                        }
                      }
                    }
                  }
                }
                frame "status2" {
                  n194 = while {
                    tunnel: [T9."wait"] -> w361
                    stop <- "删除完成 2" stop-if-true
                    n195 = event shown="[1] \"查看标注\": 鼠标按下" {
                      selector: _ -> [_ _]
                      dyn-events: _ -> [_ _]
                      timeout: 50 -> [_ _]
                      event Timeout {
                        n196 = event-data() -> ()  [unwired: 1 in, 3 out]
                      }
                      event "查看标注": Mouse Down {
                        n197 = event-data() -> ()  [unwired: 1 in, 8 out]
                        n198 = local read "穿透图原始路径"() -> (w375:path)
                        n199 = local read "临界面积百分比值"() -> (w372:dbl)
                        n200 = local read "部位信息"() -> (w377:string[])
                        n201 = local read "临界Z值"() -> (w373:i32)
                        n202 = local read "产品规格"() -> (w376:cluster{"产品长度（周长）（mm）":dbl, "产品宽度（母线长）（mm）":dbl})
                        n203 = local read "灰度阈值"() -> (w371:dbl)
                        n204 = local read "框组"() -> (w374:T3)
                        n205 = call "输入选择框号"() -> ("框号"=w378:dbl)  [unwired: 17 in, 2 out]
                        n206 = call "子界面-查看某框-只读穿透图模式.vi"("框号"=w378, "框组"=w374, "临界Z值"=w373, "临界面积百分比值"=w372, "预先配置的灰度阈值"=w371, "穿透图原始路径"=w375, "部位信息"=w377, "产品规格"=w376) -> ()  [unwired: 10 in, 2 out]
                      }
                    }
                    n207 = Wait (ms)(milliseconds to wait=u32 100 ("毫秒倍数")) -> ()  [unwired: 1 out]
                    n208 = event shown="[1] \"删除标注\": 鼠标按下" {
                      selector: _ -> [_ _]
                      dyn-events: _ -> [_ _]
                      timeout: 50 -> [_ _]
                      event Timeout {
                        n209 = event-data() -> ()  [unwired: 1 in, 3 out]
                      }
                      event "删除标注": Mouse Down {
                        n210 = event-data() -> ()  [unwired: 1 in, 3 out]
                        n211 = call "用户输入2"() -> ("框号"=w379:dbl, "确定"=w380:bool)  [unwired: 17 in, 1 out]
                        n212 = case shown="真" w380 {
                          tunnel: w379 -> [_ w381]
                          frame False {
                            # "用户取消操作"
                          }
                          frame True {
                            n213 = stacked-sequence {
                              tunnel: w381 -> [_ w388 _]
                              frame #0 {
                                # "1. 删除所有框"
                                n214 = local read "穿透图"() -> (w382:T1)
                                n215 = call "IMAQ Clear Overlay"("Image"=w382) -> ()  [unwired: 9 in, 2 out]
                              }
                              frame #1 {
                                # "2. 删除框组中指定元素"
                                n216 = local read "部位信息"() -> (w385:string[])
                                n217 = local read "框组"() -> (w387:T3)
                                n218 = Decrement(x=w388) -> (x-1=w384:dbl)
                                n219 = Delete From Array(array=w385, index=w384) -> (array with subset deleted=w383:string[])  [unwired: 1 in, 1 out]
                                n220 = Delete From Array(array=w387, index=w384) -> (array with subset deleted=w386:T3)  [unwired: 1 in, 1 out]
                                n221 = local write "框组"(w386) -> ()
                                n222 = local write "部位信息"(w383) -> ()
                              }
                              frame #2 {
                                # "3. 重画所有框"
                                n223 = while {
                                i -> [w401]
                                stop <- w392 stop-if-true
                                n224 = local read "框组"() -> (w396:T3)
                                n225 = local read "穿透图"() -> (w400:T1)
                                n226 = Array Size(array=w396) -> (size(s)=w397:i32)
                                n227 = Index Array(array=w396, index=w401) -> (element=w391:T18)
                                n228 = Increment(x=w401) -> (x+1=w408:i32)
                                n229 = local write "框数"(w397) -> ()
                                n230 = Greater Or Equal?(x=w408, y=w397) -> (x >= y?=w392:bool)
                                n231 = call "IMAQ Overlay ROI"("ROI Descriptor"=w391, "Image"=w400) -> ("Image Out"=w406:T1)  [unwired: 8 in, 1 out]
                                n232 = Unbundle(w391) -> ("Global Rectangle"=w398:i32[])  [unwired: 1 out]
                                n233 = Number To Decimal String(number=w408) -> (decimal integer string=w393:string)  [unwired: 1 in]
                                n234 = Index Array(array=w398, index=0 ("索引")) -> (element=w403:i32)
                                n235 = Index Array(array=w398, index=1 ("索引")) -> (element=w404:i32)
                                n236 = local read "自定义字体"() -> (w390:T2)
                                n237 = Concatenate Strings(w393, "#" ("字符串")) -> (w389:string)
                                n238 = Bundle(w403, w404) -> (w394:cluster{i32, i32})  [unwired: 1 in]
                                n239 = call "IMAQ Overlay Text"("Text Color (black)"=u32 16711680, "Font, Size & Style"=w390, "String"=w389, "Origin"=w394, "Image"=w406) -> ("Image Out"=w399:T1)  [unwired: 5 in, 1 out]
                                n240 = local write "穿透图"(w399) -> ()
                                }
                              }
                            }
                          }
                        }
                      }
                    }
                  }
                  n241 = Wait (ms)(milliseconds to wait=u32 50) -> ()  [unwired: 1 out]
                }
                frame "exit" {
                  n242 = Two Button Dialog(message="请确认是否完成标注" ("消息")) -> (T button?=w411:bool)  [unwired: 2 in]
                }
              }
              n243 = local read "stop"() -> (w261:bool)
              n244 = local write "穿透图"(w262) -> ()
              n245 = Or(x=w261, y=w255) -> (x .or. y?=w258:bool)
              n246 = call <vilib>:"Application Directory.vi"() -> ()  [unwired: 1 out]
            }
          }
          frame 1 {
            # "对穿透图和反射图同时画框的分支"
            n247 = while {
              shift-right: [w427] -> _
              shift-left: _ -> [w426]
              tunnel: [w424] -> _
              tunnel: [w423] -> _
              stop <- w417 stop-if-true
              (unwired) "_" ("名称或相对路径")
              (unwired) ".docx" ("名称或相对路径")
              w422 = i32[] [2] items=["No Event"=0, "Click Event"=1, "Draw Event"=2, "Size Event"=4, "Scroll Event"=5, "Double Click Event"=8] ("Which Events")
              # "循环的方式给输入图像手动画框"
              n248 = local read "反射图"() -> (w425:T1)
              n249 = local read "穿透图"() -> (w418:T1)
              n250 = invoke on="穿透图" class="ImageControl" method="Get Last Event"("Which Events"=w422) -> ("Type"=w421:i32)  [unwired: 7 in, 7 out]
              n251 = Not Equal To 0?(x=w421) -> (x != 0?=w428:bool)
              n252 = case shown="假" w428 {
                tunnel: w418 -> [w480 w488]
                tunnel: [w480 w487] -> w424
                tunnel: "Operation" -> [_ w486]
                tunnel: [w479 w481] -> w427
                tunnel: w426 -> [w479 w485]
                tunnel: w425 -> [w478 w484]
                tunnel: [w478 w483] -> w423
                frame False {
                  n253 = Wait (ms)(milliseconds to wait=u32 50 ("毫秒倍数")) -> ()  [unwired: 1 out]
                }
                frame True {
                  n254 = property on="穿透图" class="ImageControl"() -> ("ROI"=w482:T18)  [unwired: 2 in, 2 out]
                  n255 = case shown="\"overlay rectangle\"" w486 {
                    tunnel: w488 -> [w504]
                    tunnel: w482 -> [w502]
                    tunnel: [w503] -> w487
                    tunnel: w485 -> [w501]
                    tunnel: w484 -> [w500]
                    tunnel: [w499] -> w483
                    tunnel: [w498] -> w481
                    frame "overlay rectangle" {
                      n256 = flat-sequence {
                        tunnel: w504 -> [w507]
                        tunnel: [w507] -> w497
                        tunnel: w502 -> [w509]
                        tunnel: [w509] -> w496
                        tunnel: w501 -> [w508]
                        tunnel: w500 -> [w506]
                        tunnel: [w506] -> w495
                        tunnel: [w505] -> w494
                        tunnel: w497 -> [w518]
                        tunnel: w496 -> [w517]
                        tunnel: w495 -> [w523]
                        tunnel: w494 -> [w515]
                        tunnel: [w524] -> w493
                        tunnel: [w522] -> w492
                        tunnel: [w515] -> w491
                        tunnel: [w513] -> w490
                        tunnel: [w511] -> w489
                        tunnel: w493 -> [w548]
                        tunnel: w492 -> [w547]
                        tunnel: w491 -> [w546]
                        tunnel: w490 -> [w537]
                        tunnel: w489 -> [w534]
                        tunnel: [w548] -> w503
                        tunnel: [w547] -> w499
                        tunnel: [w546] -> w498
                        frame #0 {
                          # "将当前ROI数据存入框组内"
                          n257 = Build Array (concatenate)(w508, w509) -> (w505:T3)
                          n258 = local write "框组"(w505) -> ()
                        }
                        frame #1 {
                          w520 = u32[] [15663114] ("Colors (Green)")
                          w516 = u32 16711776 ("Text Color (black)")
                          # "在反射图上对应位置画框"
                          # "在穿透图上画框"
                          # "图层名Group与“框&图层计数”变量同名，\neg：1号框对应group1"
                          # "overlay text在ROI的左上角添加计数显示"
                          # "overlay ROI代表用户手画绿色框的图层添加"
                          n259 = local read "框组"() -> (w527:T3)
                          n260 = Array Size(array=w527) -> (size(s)=w511:i32)
                          n261 = Unbundle(w517) -> ("Global Rectangle"=w530:i32[])  [unwired: 1 out]
                          n262 = Number To Decimal String(number=w511) -> (decimal integer string=w512:string)  [unwired: 1 in]
                          n263 = local write "框数"(w511) -> ()
                          n264 = Concatenate Strings(w512, "#" ("字符串")) -> (w513:string)
                          n265 = Index Array(array=w530, index=1 ("索引")) -> (element=w528:i32)
                          n266 = Index Array(array=w530, index=0 ("索引")) -> (element=w529:i32)
                          n267 = local read "自定义字体"() -> (w514:T2)
                          n268 = call "IMAQ Overlay ROI"("Colors (Green)"=w520, "Group"=w513, "ROI Descriptor"=w517, "Image"=w518) -> ("Image Out"=w531:T1)  [unwired: 6 in, 1 out]
                          n269 = call "IMAQ Overlay ROI"("Colors (Green)"=w520, "Group"=w513, "ROI Descriptor"=w517, "Image"=w523) -> ("Image Out"=w521:T1)  [unwired: 6 in, 1 out]
                          n270 = Bundle(w529, w528) -> (w519:cluster{i32, i32})  [unwired: 1 in]
                          n271 = call "IMAQ Overlay Text"("Group"=w513, "Text Color (black)"=w516, "Font, Size & Style"=w514, "String"=w513, "Origin"=w519, "Image"=w521) -> ("Image Out"=w522:T1)  [unwired: 4 in, 1 out]
                          n272 = call "IMAQ Overlay Text"("Group"=w513, "Text Color (black)"=w516, "Font, Size & Style"=w514, "String"=w513, "Origin"=w519, "Image"=w531) -> ("Image Out"=w524:T1)  [unwired: 4 in, 1 out]
                        }
                        frame #2 {
                          # "存放部位信息的1D数组，后续生成报告使用"
                          # "0：位于蒙皮部位\n1：位于筋条部位"
                          n273 = call "缺陷部位标注"() -> ("位于筋条处"=w542:bool, "位于蒙皮处"=w541:bool)  [unwired: 16 in, 2 out]
                          n274 = Build Array(w541, w542) -> (w543:bool[])
                          n275 = Boolean Array To Number(Boolean array=w543) -> (number=w544:u32)
                          n276 = local read "部位信息"() -> (w536:string[])
                          n277 = case shown="1, 默认" w544 {
                            tunnel: ["蒙皮处" ("t") "筋条处" ("t")] -> w532
                            frame 1, Default {
                            }
                            frame 2 {
                            }
                          }
                          n278 = Decrement(x=w534) -> (x-1=w533:i32)
                          n279 = Insert Into Array(array=w536, index=w533, new element=w532) -> (w535:string[])
                          n280 = Concatenate Strings("框号为" ("字符串"), w537, "\n", "类别为" ("字符串"), w532) -> (→"连接的字符串":string)
                          n281 = local write "部位信息"(w535) -> ()
                        }
                      }
                    }
                  }
                }
              }
              n282 = event shown="[1] \"查看标注\": 鼠标按下" {
                selector: _ -> [_ _]
                dyn-events: _ -> [_ _]
                timeout: 50 -> [_ _]
                event Timeout {
                  n283 = event-data() -> ()  [unwired: 1 in, 3 out]
                }
                event "查看标注": Mouse Down {
                  n284 = event-data() -> ()  [unwired: 1 in, 8 out]
                  n285 = local read "反射图原始路径"() -> (w469:path)
                  n286 = local read "穿透图原始路径"() -> (w470:path)
                  n287 = local read "临界面积百分比值"() -> (w466:dbl)
                  n288 = local read "部位信息"() -> (w472:string[])
                  n289 = local read "产品规格"() -> (w471:cluster{"产品长度（周长）（mm）":dbl, "产品宽度（母线长）（mm）":dbl})
                  n290 = local read "框组"() -> (w467:T3)
                  n291 = local read "临界Z值"() -> (w468:i32)
                  n292 = local read "灰度阈值"() -> (w465:dbl)
                  n293 = call "输入选择框号"() -> ("框号"=w473:dbl)  [unwired: 17 in, 2 out]
                  n294 = call "子界面-查看某框.vi"("框号"=w473, "框组"=w467, "临界Z值"=w468, "反射图原始路径"=w469, "临界面积百分比值"=w466, "预先配置的灰度阈值"=w465, "穿透图原始路径"=w470, "部位信息"=w472, "产品规格"=w471) -> ()  [unwired: 9 in, 2 out]
                }
              }
              n295 = event shown="[1] \"删除标注\": 鼠标按下" {
                selector: _ -> [_ _]
                dyn-events: _ -> [_ _]
                timeout: 50 -> [_ _]
                event Timeout {
                  n296 = event-data() -> ()  [unwired: 1 in, 3 out]
                }
                event "删除标注": Mouse Down {
                  n297 = event-data() -> ()  [unwired: 1 in, 3 out]
                  n298 = call "用户输入"() -> ("框号"=w431:dbl, "确定"=w430:bool)  [unwired: 17 in, 1 out]
                  n299 = case shown="真" w430 {
                    tunnel: w431 -> [_ w432]
                    frame False {
                      # "用户取消操作"
                    }
                    frame True {
                      n300 = stacked-sequence {
                        tunnel: w432 -> [_ w435 _]
                        frame #0 {
                          # "1. 删除所有框"
                          n301 = local read "穿透图"() -> (w433:T1)
                          n302 = local read "反射图"() -> (w434:T1)
                          n303 = call "IMAQ Clear Overlay"("Image"=w434) -> ()  [unwired: 9 in, 2 out]
                          n304 = call "IMAQ Clear Overlay"("Image"=w433) -> ()  [unwired: 9 in, 2 out]
                        }
                        frame #1 {
                          # "2. 删除框组中指定元素"
                          n305 = local read "部位信息"() -> (w438:string[])
                          n306 = local read "框组"() -> (w440:T3)
                          n307 = Decrement(x=w435) -> (x-1=w437:dbl)
                          n308 = Delete From Array(array=w440, index=w437) -> (array with subset deleted=w439:T3)  [unwired: 1 in, 1 out]
                          n309 = Delete From Array(array=w438, index=w437) -> (array with subset deleted=w436:string[])  [unwired: 1 in, 1 out]
                          n310 = local write "框组"(w439) -> ()
                          n311 = local write "部位信息"(w436) -> ()
                        }
                        frame #2 {
                          # "3. 重画所有框"
                          n312 = while {
                            i -> [w455]
                            stop <- w444 stop-if-true
                            n313 = local read "框组"() -> (w448:T3)
                            n314 = local read "反射图"() -> (w449:T1)
                            n315 = local read "穿透图"() -> (w454:T1)
                            n316 = Array Size(array=w448) -> (size(s)=w451:i32)
                            n317 = Index Array(array=w448, index=w455) -> (element=w443:T18)
                            n318 = Increment(x=w455) -> (x+1=w464:i32)
                            n319 = local write "框数"(w451) -> ()
                            n320 = Greater Or Equal?(x=w464, y=w451) -> (x >= y?=w444:bool)
                            n321 = call "IMAQ Overlay ROI"("ROI Descriptor"=w443, "Image"=w449) -> ("Image Out"=w457:T1)  [unwired: 8 in, 1 out]
                            n322 = call "IMAQ Overlay ROI"("ROI Descriptor"=w443, "Image"=w454) -> ("Image Out"=w462:T1)  [unwired: 8 in, 1 out]
                            n323 = Unbundle(w443) -> ("Global Rectangle"=w452:i32[])  [unwired: 1 out]
                            n324 = Number To Decimal String(number=w464) -> (decimal integer string=w445:string)  [unwired: 1 in]
                            n325 = Index Array(array=w452, index=0 ("索引")) -> (element=w459:i32)
                            n326 = Index Array(array=w452, index=1 ("索引")) -> (element=w460:i32)
                            n327 = local read "自定义字体"() -> (w442:T2)
                            n328 = Concatenate Strings(w445, "#" ("字符串")) -> (w441:string)
                            n329 = Bundle(w459, w460) -> (w446:cluster{i32, i32})  [unwired: 1 in]
                            n330 = call "IMAQ Overlay Text"("Text Color (black)"=u32 16711680, "Font, Size & Style"=w442, "String"=w441, "Origin"=w446, "Image"=w457) -> ("Image Out"=w450:T1)  [unwired: 5 in, 1 out]
                            n331 = call "IMAQ Overlay Text"("Text Color (black)"=u32 16711680, "Font, Size & Style"=w442, "String"=w441, "Origin"=w446, "Image"=w462) -> ("Image Out"=w453:T1)  [unwired: 5 in, 1 out]
                            n332 = local write "反射图"(w450) -> ()
                            n333 = local write "穿透图"(w453) -> ()
                          }
                        }
                      }
                    }
                  }
                }
              }
              n334 = case shown="真" "完成标注" {
                tunnel: [FALSE ("T button?") w476] -> w414
                frame False {
                }
                frame True {
                  n335 = Two Button Dialog(message="请确认是否完成标注" ("消息")) -> (T button?=w476:bool)  [unwired: 2 in]
                }
              }
              n336 = local write "穿透图"(w424) -> ()
              n337 = local write "反射图"(w423) -> ()
              n338 = local read "stop"() -> (w420:bool)
              n339 = Or(x=w420, y=w414) -> (x .or. y?=w417:bool)
              n340 = call <vilib>:"Application Directory.vi"() -> ()  [unwired: 1 out]
            }
          }
        }
      }
      event "查看标注": Value Change {
        # "查看指定框的详细信息，包括灰度和面积阈值分割后的结果，提取到的长宽面积等信息"
        n341 = event-data() -> ()  [unwired: 1 in, 6 out]
        n342 = local read "模式选择"() -> (w562:u16)
        n343 = local read "临界面积百分比值"() -> (w554:dbl)
        n344 = local read "穿透图原始路径"() -> (w559:path)
        n345 = local read "临界Z值"() -> (w555:i32)
        n346 = local read "灰度阈值"() -> (w551:dbl)
        n347 = local read "部位信息"() -> (w561:string[])
        n348 = local read "产品规格"() -> (w560:cluster{"产品长度（周长）（mm）":dbl, "产品宽度（母线长）（mm）":dbl})
        n349 = local read "框组"() -> (w556:T3)
        n350 = call "输入选择框号"() -> ("框号"=w558:dbl, "确定"=w557:bool)  [unwired: 17 in, 1 out]
        n351 = case shown="1" w562 {
          tunnel: w561 -> [w572 w596]
          tunnel: w560 -> [w571 w595]
          tunnel: w559 -> [w570 w594]
          tunnel: w558 -> [w569 w593]
          tunnel: w557 -> [w573 w592]
          tunnel: w556 -> [w568 w591]
          tunnel: w555 -> [w567 w590]
          tunnel: w554 -> [w566 w589]
          tunnel: [w563 w588] -> w553
          tunnel: [w564 w587] -> w552
          tunnel: w551 -> [w565 w586]
          frame 0, Default {
            # "只读穿透图的图像处理方法"
            n352 = case shown="真" w573 {
              tunnel: w572 -> [_ w585]
              tunnel: w571 -> [_ w584]
              tunnel: w570 -> [_ w576]
              tunnel: w569 -> [_ w583]
              tunnel: w568 -> [_ w582]
              tunnel: w567 -> [_ w581]
              tunnel: w566 -> [_ w580]
              tunnel: w565 -> [_ w579]
              tunnel: [w575 w578] -> w564
              tunnel: [w574 w577] -> w563
              frame False {
                n353 = local read "分层类检测结果"() -> (w575:string[][])
                n354 = local read "弥散类检测结果"() -> (w574:string[][])
              }
              frame True {
                n355 = call "子界面-查看某框-只读穿透图模式.vi"("框号"=w583, "框组"=w582, "临界Z值"=w581, "临界面积百分比值"=w580, "预先配置的灰度阈值"=w579, "穿透图原始路径"=w576, "部位信息"=w585, "产品规格"=w584) -> ("弥散类检测结果"=w577:string[][], "分层类检测结果"=w578:string[][])  [unwired: 10 in]
              }
            }
          }
          frame 1 {
            # "穿透图和反射图结合的图像处理方法"
            n356 = local read "反射图原始路径"() -> (w597:path)
            n357 = case shown="真" w592 {
              tunnel: w593 -> [_ w610]
              tunnel: w586 -> [_ w609]
              tunnel: w595 -> [_ w608]
              tunnel: w596 -> [_ w607]
              tunnel: w594 -> [_ w601]
              tunnel: w597 -> [_ w600]
              tunnel: w591 -> [_ w606]
              tunnel: w590 -> [_ w605]
              tunnel: w589 -> [_ w604]
              tunnel: [w598 w603] -> w588
              tunnel: [w599 w602] -> w587
              frame False {
                # "用户取消操作"
                n358 = local read "弥散类检测结果"() -> (w598:string[][])
                n359 = local read "分层类检测结果"() -> (w599:string[][])
              }
              frame True {
                n360 = call "子界面-查看某框.vi"("框号"=w610, "框组"=w606, "临界Z值"=w605, "反射图原始路径"=w600, "临界面积百分比值"=w604, "预先配置的灰度阈值"=w609, "穿透图原始路径"=w601, "部位信息"=w607, "产品规格"=w608) -> ("弥散类检测结果"=w603:string[][], "分层类检测结果"=w602:string[][])  [unwired: 9 in]
              }
            }
          }
        }
        "弥散类检测结果" <- w553
        "分层类检测结果" <- w552
      }
      event "生成评定结果": Value Change {
        # "最终检测结果全部合并 导入word中"
        # "相当于“查看标注”一栏中的操作做循环，遍历所有框，\n将输出结果叠加为数组，作为最终结果输出并导入word"
        n361 = event-data() -> ()  [unwired: 1 in, 6 out]
        n362 = local read "分层类检测结果合并"() -> (w624:string[][])
        n363 = local read "弥散类检测结果合并"() -> (w622:string[][])
        n364 = local read "模式选择"() -> (w632:u16)
        n365 = local read "临界面积百分比值"() -> (w625:dbl)
        n366 = local read "穿透图原始路径"() -> (w629:path)
        n367 = local read "灰度阈值"() -> (w623:dbl)
        n368 = local read "临界Z值"() -> (w626:i32)
        n369 = local read "部位信息"() -> (w631:string[])
        n370 = local read "产品规格"() -> (w630:cluster{"产品长度（周长）（mm）":dbl, "产品宽度（母线长）（mm）":dbl})
        n371 = local read "框组"() -> (w628:T3)
        n372 = local read "框数"() -> (w627:dbl)
        n373 = case shown="1" w632 {
          tunnel: [w641 w676] -> w636
          tunnel: [w639 w666] -> w635
          tunnel: w631 -> [w649 w675]
          tunnel: w630 -> [w647 w674]
          tunnel: w629 -> [w646 w673]
          tunnel: w628 -> [w645 w672]
          tunnel: w627 -> [w648 w671]
          tunnel: w623 -> [_ w670]
          tunnel: w626 -> [w644 w669]
          tunnel: w625 -> [w643 w668]
          tunnel: w624 -> [w640 w667]
          tunnel: w623 -> [w642 _]
          tunnel: w622 -> [w638 w665]
          frame 0, Default {
            # "只读穿透图的图像处理方法"
            n374 = for {
              N: w648 -> [_]
              tunnel: w649 -> [w664]
              tunnel: w647 -> [w663]
              tunnel: w646 -> [w650]
              tunnel: w645 -> [w662]
              tunnel: w644 -> [w661]
              tunnel: w643 -> [w660]
              tunnel: w642 -> [w659]
              shift-right: [w657] -> w641
              shift-left: w640 -> [w656]
              shift-right: [w651] -> w639
              shift-left: w638 -> [w652]
              i -> [w655]
              n375 = Increment(x=w655) -> (x+1=w654:i32)
              n376 = call "子界面-查看某框-不显示界面-只读穿透图模式.vi"("框号"=w654, "框组"=w662, "临界Z值"=w661, "临界面积百分比值"=w660, "预先配置的灰度阈值"=w659, "穿透图原始路径"=w650, "部位信息"=w664, "产品规格"=w663) -> ("弥散类检测结果"=w653:string[][], "分层类检测结果"=w658:string[][])  [unwired: 10 in]
              n377 = Build Array (concatenate)(w652, w653) -> (w651:string[][])
              n378 = Build Array (concatenate)(w656, w658) -> (w657:string[][])
            }
          }
          frame 1 {
            # "穿透图和反射图结合的图像处理方法"
            n379 = local read "反射图原始路径"() -> (w677:path)
            n380 = for {
              N: w671 -> [_]
              tunnel: w677 -> [w678]
              shift-right: [w683] -> w676
              shift-left: w667 -> [w685]
              tunnel: w675 -> [w693]
              tunnel: w674 -> [w692]
              tunnel: w673 -> [w679]
              tunnel: w672 -> [w691]
              tunnel: w670 -> [w690]
              tunnel: w669 -> [w689]
              tunnel: w668 -> [w688]
              shift-right: [w682] -> w666
              shift-left: w665 -> [w680]
              i -> [w687]
              n381 = Increment(x=w687) -> (x+1=w686:i32)
              n382 = call "子界面-查看某框-不显示界面.vi"("框号"=w686, "框组"=w691, "临界Z值"=w689, "反射图原始路径"=w678, "临界面积百分比值"=w688, "预先配置的灰度阈值"=w690, "穿透图原始路径"=w679, "部位信息"=w693, "产品规格"=w692) -> ("弥散类检测结果"=w681:string[][], "分层类检测结果"=w684:string[][])  [unwired: 9 in]
              n383 = Build Array (concatenate)(w685, w684) -> (w683:string[][])
              n384 = Build Array (concatenate)(w680, w681) -> (w682:string[][])
            }
          }
        }
        n385 = local write "弥散类检测结果合并"(w635) -> ()
        n386 = local write "分层类检测结果合并"(w636) -> ()
        n387 = flat-sequence {
          tunnel: w635 -> [w694]
          tunnel: w636 -> [w695]
          tunnel: [w695] -> w614
          tunnel: [w694] -> w612
          tunnel: w614 -> [w736]
          tunnel: [w736] -> w613
          tunnel: w612 -> [w735]
          tunnel: [w735] -> w611
          tunnel: w613 -> [w743]
          tunnel: w611 -> [w742]
          tunnel: [w743] -> w621
          tunnel: [w742] -> w620
          tunnel: [w741] -> w618
          tunnel: [w740] -> w617
          tunnel: [w763] -> w634
          tunnel: [w762] -> w633
          tunnel: w621 -> [w753]
          tunnel: w620 -> [w756]
          tunnel: [w756] -> w619
          tunnel: w618 -> [w755]
          tunnel: w617 -> [w754]
          tunnel: w634 -> [w774]
          tunnel: w633 -> [w773]
          tunnel: w619 -> [w772]
          tunnel: [w771] -> w616
          tunnel: [w770] -> w615
          tunnel: w616 -> [w790]
          tunnel: w615 -> [w789]
          frame #0 {
            n388 = while {
              tunnel: [w702] -> _
              i -> [w706]
              stop <- w702 stop-if-true
              w711 = 1 items=["White", "Black", "Inverted", "Black on White", "White on Black"] ("Color")
              w715 = u16 2 items=["Frame", "Paint", "Invert Frame", "Invert Paint"] ("Draw Mode")
              w708 = u16 1 items=["Line", "Rectangle", "Oval"] ("Shape to draw")
              # "生成绘制了ROI的图像\n可以用于后续的图片导出保存"
              n389 = local read "框组"() -> (w705:T3)
              n390 = local read "穿透图"() -> (w698:T1)
              n391 = Array Size(array=w705) -> (size(s)=w723:i32)
              n392 = local read "ROImask"() -> (w697:T1)
              n393 = Index Array(array=w705, index=w706) -> (element=w704:T18)
              n394 = Unbundle(w704) -> ("Global Rectangle"=w703:i32[])  [unwired: 1 out]
              n395 = Increment(x=w706) -> (x+1=w724:i32)
              n396 = Greater Or Equal?(x=w724, y=w723) -> (x >= y?=w702:bool)
              n397 = Index Array(array=w703, index=0 ("索引")) -> (element=w713:i32)
              n398 = Index Array(array=w703, index=2 ("索引")) -> (element=w718:i32)
              n399 = Index Array(array=w703, index=1 ("索引")) -> (element=w712:i32)
              n400 = Index Array(array=w703, index=3 ("索引")) -> (element=w717:i32)
              n401 = Number To Decimal String(number=w724) -> (decimal integer string=w709:string)  [unwired: 1 in]
              n402 = Build Array(w713, w712, w718, w717) -> (w699:i32[])
              n403 = call "IMAQ Draw"("Draw Mode"=w715, "Shape to draw"=w708, "Pixel Color"=sgl 0.0, "Coordinates"=w699, "Image Src"=w698) -> ("Image Dst Out"=w714:T1)  [unwired: 5 in, 1 out]
              n404 = Concatenate Strings(w709, "#" ("字符串")) -> (w707:string)
              n405 = local read "自定义字体"() -> (w700:T2)
              n406 = Build Array(w713, w712) -> (w701:i32[])
              n407 = call "IMAQ Draw Text"("String"=w707, "Insertion Point"=w701, "Color"=w711, "Font, Size & Style"=w700, "Image Dst"=w697, "Image Src"=w714) -> ("Image Dst Out"=w696:T1)  [unwired: 2 in, 3 out]
              "ROImask" <- w696
              n408 = local write "ROImask"(w696) -> ()
            }
          }
          frame #1 {
            n409 = local read "穿透图原始路径"() -> (w734:path)
            n410 = local read "ROImask"() -> (w725:T1)
            n411 = Path To String(path=w734) -> (string=w731:string)
            n412 = String Length(string=w731) -> (length=w732:i32)
            n413 = Subtract(x=w732, y=4) -> (x-y=w733:i32)
            n414 = Replace Substring(3:w733, 4:"_标注后.png" ("字符串"), 5:w731) -> (1:w730:string)  [unwired: 1 in, 1 out]
            n415 = String To Path(string=w730) -> (path=w726:path)
            "标注后的图片路径" <- w726
            n416 = call-poly "IMAQ Write File 2"("Image Quality"=u32 1000, "File Path"=w726, "Image"=w725) -> ()  [unwired: 7 in, 2 out]
          }
          frame #2 {
            n417 = call <vilib>:"Application Directory.vi"() -> ("Application Directory"=w739:path)
            n418 = Build Path(base path=w739, name or relative path="report-template.docx") -> (appended path=w737:path)
            n419 = call <vilib>:"Create Report.vi"("window state (normal)"=T10."maximized", "report type"=Report_Type."Word", "template (empty)"=w737) -> ("report out"=w741:refnum<class "NI_report.lvclass">, "error out"=w740:errorcluster)  [unwired: 11 in]
          }
          frame #3 {
            n420 = Get Date/Time String(date format (0)=enum16{"short", "long", "abbreviated"}."long" ("日期格式(0)")) -> (date string=w760:string, time string=w761:string)  [unwired: 2 in]
            n421 = local read "标注后的图片路径"() -> (w751:path)
            n422 = Concatenate Strings(w760, w761) -> (w759:string)
            n423 = call-poly <vilib>:"Append Report Text.vi"("report in"=w755, "MS Office parameters"=T14 {"position (excel)"={"row"=0, "column"=0}, "name (excel)"="", "bookmark (word)"="time"}, "text"=w759, "error in (no error)"=w754) -> ("report out"=w750:refnum<class "NI_report.lvclass">, "error out"=w748:errorcluster)  [unwired: 8 in, 2 out]
            n424 = call-poly <vilib>:"Append Image to Report.vi"("report in"=w750, "alignment (default)"=HTML_Report_Image_Alignment."MIDDLE", "MS Office parameters"=T13 {"position (Excel)"={"row"=0, "column"=0}, "name (Excel)"="", "bookmark (Word)"="image"}, "path or URL of image"=w751, "error in (no error)"=w748) -> ("report out"=w747:refnum<class "NI_report.lvclass">, "error out"=w746:errorcluster)  [unwired: 7 in, 2 out]
            n425 = call <vilib>:"Word Easy Text.vi"("report in"=w747, "text"="分层类", "alignment (left)"=enum16{"Left", "Centered", "Right", "Justify"}."Left", "font"=T15 {"font name"="", "font size"=0.0, "bold"=0, "italic"=0, "underline"=0, "strike through"=0, "font color"=16777216}, "error in (no error)"=w746) -> ("report out"=w765:refnum<class "NI_report.lvclass">, "error out"=w766:errorcluster)  [unwired: 8 in, 1 out]
            n426 = call-poly <vilib>:"Word Easy Table.vi"("report in"=w765, "column headers"=string[] ["框号", "长/mm", "宽/mm", "面积/mm2", "Z值/mm", "部位", "类型", "合格性"], "data"=w753, "error in (no error)"=w766) -> ("report out"=w763:refnum<class "NI_report.lvclass">, "error out"=w762:errorcluster)  [unwired: 9 in, 1 out]
          }
          frame #4 {
            n427 = call <vilib>:"Word Easy Text.vi"("report in"=w774, "text"="弥散类", "alignment (left)"=enum16{"Left", "Centered", "Right", "Justify"}."Left", "font"=T15 {"font name"="", "font size"=0.0, "bold"=0, "italic"=0, "underline"=0, "strike through"=0, "font color"=16777216}, "error in (no error)"=w773) -> ("report out"=w776:refnum<class "NI_report.lvclass">, "error out"=w777:errorcluster)  [unwired: 8 in, 1 out]
            n428 = call-poly <vilib>:"Word Easy Table.vi"("report in"=w776, "column headers"=string[] ["框号", "长/mm", "宽/mm", "面积/mm2", "Z值/mm", "部位", "类型", "合格性"], "data"=w772, "error in (no error)"=w777) -> ("report out"=w771:refnum<class "NI_report.lvclass">, "error out"=w770:errorcluster)  [unwired: 9 in, 1 out]
          }
          frame #5 {
            n429 = local read "穿透图原始路径"() -> (w781:path)
            n430 = Path To String(path=w781) -> (string=w786:string)
            n431 = String Length(string=w786) -> (length=w787:i32)
            n432 = Subtract(x=w787, y=4) -> (x-y=w788:i32)
            n433 = Replace Substring(3:w788, 4:"_.docx" ("字符串"), 5:w786) -> (1:w785:string)  [unwired: 1 in, 1 out]
            n434 = String To Path(string=w785) -> (path=w782:path)
            "添加的路径" <- w782
            n435 = call-dynamic "Save Report to File.vi"("report in"=w790, "report file path"=w782, "prompt to replace? (F)"=TRUE, "error in (no error)"=w789) -> ("report out"=w794:refnum<class "NI_report.lvclass">, "error out"=w793:errorcluster)  [unwired: 10 in]
            n436 = call <vilib>:"Word Bring to Front.vi"("report in"=w794, "window state (maximized)"=enum16{"maximized", "minimized", "normal"}."normal", "error in (no error)"=w793) -> ()  [unwired: 11 in, 2 out]
          }
          frame #6 {
            n437 = One Button Dialog(message="完成评定并退出程序！\n请查看word报告" ("消息")) -> ()  [unwired: 1 in, 1 out]
          }
        }
      }
      event "stop": Value Change {
        # "退出软件"
        n438 = event-data() -> ("NewVal"=w799:bool)  [unwired: 1 in, 4 out]
        n439 = Two Button Dialog(message="是否关闭本软件？" ("消息")) -> (T button?=w800:bool)  [unwired: 2 in]
        n440 = And(x=w799, y=w800) -> (x .and. y?=w798:bool)
        n441 = case shown="真" w798 {
          frame False {
          }
          frame True {
            w801 = TRUE ("All Images? (No)")
            n442 = local read "穿透图"() -> (w803:T1)
            n443 = local read "反射图"() -> (w802:T1)
            n444 = call "IMAQ Dispose"("All Images? (No)"=w801, "Image"=w803) -> ()  [unwired: 4 in, 1 out]
            n445 = call "IMAQ Dispose"("All Images? (No)"=w801, "Image"=w802) -> ()  [unwired: 4 in, 1 out]
            n446 = disable-structure shown="RUN_TIME_ENGINE==True" {
              frame condition #0 {
                n447 = Quit LabVIEW() -> ()  [unwired: 1 in]
              }
              frame condition #1 (active) {
                n448 = Stop() -> ()  [unwired: 1 in]
              }
            }
          }
        }
      }
    }
  }
  n449 = disable-structure shown="禁用" {
    frame Disabled {
      n450 = while {
        stop <- FALSE stop-if-true
        n451 = local read "删除标注"() -> (w807:bool)
        n452 = local read "查看标注"() -> (w806:bool)
        n453 = Or(x=w807, y=w806) -> (x .or. y?=w808:bool)
        n454 = local write "开始标注"(w808) -> ()
        n455 = Wait Until Next ms Multiple(millisecond multiple=u32 50 ("毫秒倍数")) -> ()  [unwired: 1 out]
      }
    }
    frame Enabled {
    }
  }
  "框组" <- T3 [] ("框组")
  "框数" <- 0.0 ("框数")
  "自定义字体" <- T2 {"Desired Font (Application)"=enum."User-specified Font", "[User-specified Font]"={"Font Name"="", "Size"=80, "Strikeout?"=FALSE, "Italic?"=FALSE, "Underline?"=FALSE, "Outline?"=FALSE, "Shadow?"=FALSE, "Bold?"=TRUE, "Rotation Angle"=0.0}, "Horizontal Alignment"=0, "Vertical Alignment"=0} ("Font, Size & Style")
  "部位信息" <- string[] ["", "", "", "", "", "", "", "", ""] ("部位信息")
  "分层类检测结果合并" <- string[][] [] ("弥散类检测结果合并")
  "弥散类检测结果合并" <- string[][] [] ("弥散类检测结果合并")
  "临界面积百分比值" <- w4
  "输入的灰度阈值" <- w5
